vi "H2O_DIAL_NCAR_4CH_v4.05.vi"() -> ()   [LabVIEW 2012]
uses:
  C:/Users/H2ODial/Desktop/Shared Telescope WV DIAL Code/Libraries and VIs/PowerMeterCommands.dll
  Libraries and VIs/PowerMeterCommands.dll
  <vilib>/DAQmx/write.llb/DAQmx Write (Digital 1D Bool NChan 1Samp 1Line).vi
  <vilib>/DAQmx/miscellaneous.llb/DAQmx Fill In Error Info.vi
  <vilib>/Analysis/baseanly.llb/Mean (DBL).vi
  Libraries and VIs/Scalar_Data.vi
  Libraries and VIs/Scalar_Data_3.vi
  Libraries and VIs/Scalar_Data_2.vi
  Libraries and VIs/Scalar_Data_4.vi
  <vilib>/Analysis/NI_AALBase.lvlib
  Libraries and VIs/CLDevIFace.dll
panel:
  out "FileHour":i32=21
  out "L_Count":i32=25
  out "sigma_off_total":dbl[](array[numeric])=[5.235525125067343e-25, 5.206358319245337e-25, 5.177318750524933e-25, 5.148406424862825e-25, 5.119621341127451e-25, 5.090963491196627e-25, 5.062432860011865e-25, 5.034029425635027e-25, 5.005753159352157e-25, 4.977604025706667e-25, 4.949581982592347e-25, 4.921686981325722e-25, 4.893918966711095e-25, 4.866277877122191e-25, 4.8387636445644285e-25, 4.811376194764721e-25, 4.784115447230487e-25, 4.756981315339233e-25, 4.729973706394386e-25, 4.703092521721628e-25, 4.6763376567211625e-25, 4.6497090009594435e-25, 4.623206438225019e-25, 4.596829846622293e-25, 4.57057909862005e-25, 4.544454061150213e-25, 4.518454595652437e-25, 4.492580558158126e-25, 4.4668317993693425e-25, 4.441208164702635e-25, 4.41570949437918e-25, 4.390335623482575e-25, 4.365086382028137e-25, 4.339961595028071e-25, 4.314961082547237e-25, 4.290084659777996e-25, 4.2653321370993085e-25, 4.240703320135042e-25, 4.216198009811418e-25, 4.191816002426457e-25, 4.16755708969195e-25, 4.143421058805604e-25, 4.1194076924960845e-25, 4.095516769084665e-25, 4.0717480625238245e-25, 4.0481013424706545e-25, 4.0245763743206737e-25, 4.001172919260011e-25, 3.977890734322512e-25, 3.9547295724256756e-25, 3.931689182419048e-25, 3.908769309139365e-25, 3.8859696934393876e-25, 3.863290072236815e-25, 3.840730178557474e-25, 3.8182897415734565e-25, 3.7959684866403156e-25, 3.773766135338825e-25, 3.7516824055099053e-25, 3.729717011286995e-25, 3.707869663137923e-25, 3.686140067893342e-25, 3.664527928779591e-25, 3.643032945453827e-25, 3.621654814033011e-25, 3.600393227122229e-25, 3.579247873843723e-25, 3.5582184398664743e-25, 3.5373046074361216e-25, 3.5165060553938904e-25, 3.4958224592064764e-25, 3.475253490990589e-25, 3.454798819536632e-25, 3.4344581103303625e-25, 3.414231025576395e-25, 3.394117224218377e-25, 3.37411636196096e-25, 3.3542280912885406e-25, 3.3344520614845767e-25, 3.3147879186525413e-25, 3.295235305730259e-25, 3.275793862509532e-25, 3.2564632256504646e-25, 3.237243028702917e-25, 3.2181329021119735e-25, 3.1991324732434905e-25, 3.180241366390581e-25, 3.161459202790299e-25, 3.142785600633377e-25, 3.1242201750825597e-25, 3.1057625382770893e-25, 3.0874122993477767e-25, 3.0691690644282785e-25, 3.051032436660927e-25, 3.0330020162078266e-25, 3.0150774002602592e-25, 2.997258183045521e-25, 2.979543955833093e-25, 2.961934306943937e-25, 2.944428821752431e-25, 2.9270270826932477e-25, 2.909728669267514e-25, 2.8925331580414936e-25, 2.875440122654977e-25, 2.8584491338173137e-25, 2.841559759313169e-25, 2.8247715639976386e-25, 2.80808410980223e-25, 2.791496955724979e-25, 2.775009657833479e-25, 2.7586217692567447e-25, 2.742332840183121e-25, 2.7261424178518227e-25, 2.710050046547509e-25, 2.6940552675881075e-25, 2.6781576193155516e-25, 2.6623566370876434e-25, 2.646651853260364e-25, 2.6310427971768174e-25, 2.615528995144771e-25, 2.600109970428841e-25, 2.5847852432207883e-25, 2.569554330624564e-25, 2.554416746633416e-25, 2.5393720020962457e-25, 2.5244196047033826e-25, 2.5095590589459477e-25, 2.4947898660936654e-25, 2.480111524155541e-25, 2.4655235278440513e-25, 2.451025368544176e-25, 2.436616534266772e-25, 2.422296509605852e-25, 2.408064775697375e-25, 2.3939208101763006e-25, 2.3798640871112015e-25, 2.365894076971971e-25, 2.352010246556833e-25, 2.3382120589521406e-25, 2.324498973455175e-25, 2.3108704455300754e-25, 2.2973259267270024e-25, 2.283864864626908e-25, 2.270486702764721e-25, 2.257190880557015e-25, 2.2439768332388837e-25, 2.2308439917739663e-25, 2.2177917827749597e-25, 2.20481962844103e-25, 2.19192694645104e-25, 2.179113149897461e-25, 2.166377647190967e-25, 2.153719841983278e-25, 2.1411391330535246e-25, 2.1286349142540036e-25, 2.1162065743868337e-25, 2.103853497130775e-25, 2.091575060946101e-25, 2.079370638983031e-25, 2.0672395989815037e-25, 2.0551813031976677e-25, 2.0431951082869756e-25, 2.0312803652523447e-25, 2.019436419319984e-25, 2.0076626098781596e-25, 1.9959582703908636e-25, 1.9843227283026113e-25, 1.9727553050009988e-25, 1.9612553156963306e-25, 1.9498220693936616e-25, 1.9384548688025462e-25, 1.9271530103114487e-25, 1.915915783921294e-25, 1.9047424731896738e-25, 1.8936323552292957e-25, 1.8825847006561212e-25, 1.8715987735714719e-25, 1.8606738315918164e-25, 1.8498091257941087e-25, 1.8390039007904753e-25, 1.8282573946936752e-25, 1.8175688392200846e-25, 1.80693745969556e-25, 1.7963624751388698e-25, 1.7858430983630522e-25, 1.7753785360393623e-25, 1.7649679888396773e-25, 1.7546106515613228e-25, 1.7443057132789558e-25, 1.7340523575155863e-25, 1.723849762422857e-25, 1.7136971010131167e-25, 1.7035935413825008e-25, 1.6935382469544605e-25, 1.6835303767796407e-25, 1.6735690858143057e-25, 1.6636535252563445e-25, 1.653782842907513e-25, 1.643956183497921e-25, 1.6341726891478545e-25, 1.624431499756322e-25, 1.6147317534796005e-25, 1.6050725871551994e-25, 1.5954531368896971e-25, 1.585872538492723e-25, 1.576329928151117e-25, 1.566824442883223e-25, 1.5573552212546758e-25, 1.5479214039898043e-25, 1.5385221346219397e-25, 1.5291565602013113e-25, 1.519823831962039e-25, 1.5105231061650234e-25, 1.5012535447460145e-25, 1.49201431624485e-25, 1.482804596459418e-25, 1.4736235693849326e-25, 1.46447042805166e-25, 1.455344375360034e-25, 1.4462446250285657e-25, 1.4371704024629248e-25, 1.4281209456557682e-25, 1.4190955061389853e-25, 1.410093350012645e-25, 1.4011137586880333e-25, 1.3921560301221658e-25, 1.3832194795253431e-25, 1.3743034404767374e-25, 1.3654072658699072e-25, 1.3565303288298996e-25, 1.3476720236918642e-25, 1.3388317669734332e-25, 1.3300089982893968e-25, 1.3212031812258562e-25, 1.3124138043688156e-25, 1.3036403820696332e-25, 1.2948824553577423e-25, 1.2861395928315612e-25, 1.2774113913410786e-25, 1.2686974768684636e-25, 1.2599975053009544e-25, 1.2513111630057894e-25, 1.2426381676023619e-25, 1.2339782685325752e-25, 1.2253312476934588e-25, 1.2166969199403071e-25, 1.2080751335374065e-25, 1.1994657705541538e-25, 1.1908687474046665e-25, 1.182284014933639e-25, 1.1737115587808914e-25, 1.1651513996305814e-25, 1.1566035931942852e-25, 1.1480682304187532e-25, 1.1395454373665928e-25, 1.1310353751750977e-25, 1.1225382399779688e-25, 1.1140542626706877e-25, 1.1055837085176348e-25, 1.097126877076807e-25, 1.0886841014622313e-25, 1.0802557481625692e-25, 1.07184221622742e-25, 1.0634439369229237e-25, 1.0550613727868173e-25, 1.0466950171251473e-25, 1.038345393031225e-25, 1.0300130526116006e-25, 1.0216985760646603e-25, 1.0134025706453978e-25, 1.0051256696943142e-25, 9.968685315566847e-26, 9.886318383691271e-26, 9.804162950309608e-26, 9.722226278487634e-26, 9.640515833439737e-26, 9.559039270504641e-26]
  out "sigma_on_total":dbl[](array[numeric])=[2.04144506552878e-23, 2.03363164868905e-23, 2.025747572591412e-23, 2.017794430211764e-23, 2.009773817105046e-23, 2.0016873309336366e-23, 1.9935365706299817e-23, 1.9853231355693705e-23, 1.977048625166467e-23, 1.9687146378445772e-23, 1.9603227705421816e-23, 1.951874618043596e-23, 1.9433717722469982e-23, 1.9348158215951184e-23, 1.9262083503317138e-23, 1.9175509380334025e-23, 1.9088451588558353e-23, 1.900092581092815e-23, 1.8912947664136064e-23, 1.882453269524831e-23, 1.8735696373998732e-23, 1.8646454089324773e-23, 1.8556821142337575e-23, 1.8466812743522004e-23, 1.837644400527498e-23, 1.8285729940141764e-23, 1.8194685453299388e-23, 1.810332533962471e-23, 1.8011664280533842e-23, 1.7919716836950586e-23, 1.7827497447925897e-23, 1.7735020425748035e-23, 1.7642299952670358e-23, 1.754935007742652e-23, 1.7456184710818656e-23, 1.736281762398895e-23, 1.726926244502896e-23, 1.717553265574508e-23, 1.7081641588579278e-23, 1.6987602425458152e-23, 1.68934281932253e-23, 1.6799131763488586e-23, 1.6704725849056047e-23, 1.6610223002991386e-23, 1.6515635614647057e-23, 1.642097591109307e-23, 1.632625595307178e-23, 1.623148763389859e-23, 1.6136682679517084e-23, 1.6041852645568704e-23, 1.5947008916673987e-23, 1.585216270718842e-23, 1.5757325057977178e-23, 1.5662506836735098e-23, 1.556771873772616e-23, 1.5472971280958616e-23, 1.5378274811478395e-23, 1.5283639499771967e-23, 1.5189075341266753e-23, 1.5094592155613525e-23, 1.5000199588045791e-23, 1.4905907108522535e-23, 1.4811724011961994e-23, 1.471765941921017e-23, 1.4623722277116113e-23, 1.452992135870101e-23, 1.4436265263735662e-23, 1.4342762419712705e-23, 1.4249421083199486e-23, 1.4156249339056498e-23, 1.406325510226225e-23, 1.397044611884901e-23, 1.3877829966903115e-23, 1.378541405732157e-23, 1.3693205635246762e-23, 1.3601211780942827e-23, 1.3509439411338302e-23, 1.3417895281011788e-23, 1.3326585983534608e-23, 1.3235517953452217e-23, 1.3144697466818022e-23, 1.3054130643262744e-23, 1.2963823446919121e-23, 1.287378168942871e-23, 1.2784011028907963e-23, 1.269451697446829e-23, 1.2605304885835775e-23, 1.2516379975894178e-23, 1.2427747311540186e-23, 1.2339411817103151e-23, 1.2251378274123229e-23, 1.2163651324251236e-23, 1.2076235471304545e-23, 1.1989135081970437e-23, 1.190235438818644e-23, 1.1815897489244797e-23, 1.1729768353364932e-23, 1.1643970819286305e-23, 1.1558508598932436e-23, 1.1473385278221191e-23, 1.1388604319479822e-23, 1.1304169063843004e-23, 1.122008273184013e-23, 1.1136348426833785e-23, 1.1052969135364539e-23, 1.0969947730316559e-23, 1.0887286971537587e-23, 1.0804989509475963e-23, 1.07230578850557e-23, 1.0641494533043776e-23, 1.0560301782926725e-23, 1.047948186150434e-23, 1.0399036894250036e-23, 1.031896890763079e-23, 1.0239279830219628e-23, 1.0159971494762414e-23, 1.0081045640686342e-23, 1.0002503914953993e-23, 9.924347874544637e-24, 9.846578987076846e-24, 9.7691986343937e-24, 9.692208112477475e-24, 9.615608634312278e-24, 9.53940133157985e-24, 9.463587255028901e-24, 9.388167378138146e-24, 9.313142597016321e-24, 9.238513733351717e-24, 9.164281535166715e-24, 9.090446678433916e-24, 9.017009769507337e-24, 8.943971345840847e-24, 8.871331877547395e-24, 8.799091769345933e-24, 8.727251362469196e-24, 8.655810934528908e-24, 8.584770703015792e-24, 8.514130824937205e-24, 8.443891399845548e-24, 8.374052469666215e-24, 8.30461402165979e-24, 8.23557598842531e-24, 8.166938250220636e-24, 8.09870063571327e-24, 8.03086292329742e-24, 7.963424843129024e-24, 7.896386077455162e-24, 7.829746261877174e-24, 7.76350498767362e-24, 7.697661801548124e-24, 7.63221620790868e-24, 7.567167669492106e-24, 7.502515609040041e-24, 7.438259409201822e-24, 7.374398415389291e-24, 7.310931935299025e-24, 7.247859240849607e-24, 7.18517956905468e-24, 7.122892123050664e-24, 7.060996072777461e-24, 6.99949055663218e-24, 6.938374681458788e-24, 6.877647524805744e-24, 6.8173081345645e-24, 6.757355530696846e-24, 6.697788705968921e-24, 6.638606626367178e-24, 6.579808233049281e-24, 6.521392441796805e-24, 6.463358144925488e-24, 6.4057042113363034e-24, 6.3484294880639726e-24, 6.291532800599893e-24, 6.23501295336718e-24, 6.178868731199306e-24, 6.123098899483674e-24, 6.067702204884087e-24, 6.01267737674528e-24, 5.958023126645283e-24, 5.903738150186674e-24, 5.849821126538989e-24, 5.7962707201795e-24, 5.743085580692951e-24, 5.6902643436582656e-24, 5.637805631506092e-24, 5.585708053569947e-24, 5.533970207051788e-24, 5.482590677443224e-24, 5.431568039066743e-24, 5.380900855603735e-24, 5.3305876804860644e-24, 5.2806270576492845e-24, 5.231017521895454e-24, 5.1817575992506746e-24, 5.132845807674582e-24, 5.084280657272612e-24, 5.036060650860678e-24, 4.988184284511523e-24, 4.940650047510622e-24, 4.893456423348436e-24, 4.846601889770117e-24, 4.8000849193904994e-24, 4.753903979624906e-24, 4.7080575337261334e-24, 4.662544040368925e-24, 4.617361954873326e-24, 4.572509728567645e-24, 4.5279858098761176e-24, 4.4837886444191376e-24, 4.4399166752196636e-24, 4.396368343110522e-24, 4.353142086723786e-24, 4.310236343387402e-24, 4.267649548693646e-24, 4.225380137567508e-24, 4.1834265436346086e-24, 4.141787200071118e-24, 4.100460539746925e-24, 4.059444995273427e-24, 4.018738999519791e-24, 3.978340985645206e-24, 3.9382493872264135e-24, 3.898462638564106e-24, 3.858979175244214e-24, 3.81979743343543e-24, 3.7809158512434734e-24, 3.742332867827665e-24, 3.704046924201295e-24, 3.666056463311095e-24, 3.628359930032478e-24, 3.590955771418263e-24, 3.553842436936342e-24, 3.517018378534459e-24, 3.480482050624481e-24, 3.444231910627635e-24, 3.4082664187032186e-24, 3.372584038041973e-24, 3.3371832351443385e-24, 3.3020624795514383e-24, 3.2672202442735406e-24, 3.2326550059709053e-24, 3.1983652446833905e-24, 3.164349444235738e-24, 3.130606092186823e-24, 3.0971336800695645e-24, 3.06393070340578e-24, 3.030995661721895e-24, 2.9983270585653876e-24, 2.9659234019996817e-24, 2.933783204123355e-24, 2.9019049814229044e-24, 2.870287254971944e-24, 2.8389285501614312e-24, 2.8078273970940295e-24, 2.7769823303790683e-24, 2.746391889257262e-24, 2.7160546177804717e-24, 2.6859690647949184e-24, 2.65613378374283e-24, 2.6265473332620553e-24, 2.597208276553025e-24, 2.568115182026435e-24, 2.5392666228001165e-24, 2.510661177266997e-24, 2.48229742859929e-24, 2.454173965243289e-24, 2.4262893806011815e-24, 2.3986422732292233e-24, 2.371231246858978e-24, 2.344054910309026e-24, 2.3171118776147202e-24, 2.2904007680434033e-24, 2.2639202059521634e-24, 2.237668821064949e-24, 2.211645248222906e-24, 2.185848127501672e-24, 2.16027610436914e-24]
  out "background start":u32=269
  in  "Tab Control 2":enum32{"WV ND far", "WV ND near"}(tab)
  out "Water Vapor Number Density":dbl[][](graph)=[[1.7566467714554592, 1.7112237483974937, 1.6748749506264644, 1.5531626763016915, 1.4925818532745008, 1.4691395321648246, 1.3246167272218103, 1.2269868164425828, 1.3255222864560143, 1.4516476142332622, 1.4317488856306848, 1.4006762178952012, 1.3734771433422062, 1.3434494748177286, 1.3451253921115185, 1.1715664766487153, 0.9603460494298136, 1.167803410589512, 1.5837995618115461, 1.4928182826946899, 0.7830880837201466, 0.7124646182150762, 1.5821683844017884, 1.897616667905768, 1.3567387444432506, 0.7685875264908889, 0.8821075379606124, 0.9580561941866925, 0.6860769280953256, 0.9548855995658682, 0.34317959293560385, -0.48852203085720447, 0.4000953836211541, 1.6276766516112087, 0.6582217273425924, -0.3701431622041616, 0.5624402493727769, 1.5020315964518778, 1.9490328819529277, 0.5687081180809571, 0.14829866816328646, 0.15078097843341215, -0.4052462468388696, 0.00726247689994212, 0.6405048350399107, 1.070833208753949, 1.2895427721533483, 0.4806362739895196, 1.0023443102054248, 1.0632416785543921, 0.5419834758759072, 1.216133517204536, 2.9403717140528025, 6.026761955773755, 2.4631218194880327, -0.5616309456927226, -2.1863539244969585, -1.1172913943803293, -0.5764679216345628, -0.32669650897300184, 1.367021471278265, 1.8114322755592884, 5.333676793891489, -0.6746298517642445, 0.2493668025284435, -0.968407653253325, -1.2597627805763916, -0.873029286367304, 0.03600152424325076, -0.4128660335725368, -1.9925424606024094, -4.686321918196433, -9.773012324862892, 8.321919527003791, -3.3327600174211867, -2.2694378626967384, -0.7880407452058662, -3.126604726748548, 4.237818794739943, 1.9339834290875324, -0.5031068702025436, 2.834157585206886, 1.9194876875375615, -7.621882484032893, 10.053582111673641, 24.583430974758375, 1.6051353561748916, 1.9018880545441958, -2.199648496161464, -2.8171837647098044, -0.1810860182335741, -5.818897288164005, -5.390599800188094, -5.557229048352483, -11.486454195723043, -1.7389583913430502, 10.399164750341773, -1.6277519987253517, -10.371881860352497, -4.1738257491608035, 4.726765211939229, 3.4342788042530907, 1.9890722023134209, 2.4803275304917283, -3.41607671638549, -21.568626510054933, 3.388736921345587, 1.9568309789098535, -4.193155315940581, -5.703648396321129, -9.41827741518324, -0.21393347906320512, 19.9442339598812, -7.779013774001198, -17.279927512309417, -1.0627832528431156, -5.628901623765271, -15.970763810695905, -4.961662952263955, -10.607717740119206, -6.080359409806072, -4.630196687396562, -15.179266411863631, 16.998783731568285, 19.683522058787823, 4.441696343538448, 2.9936653651043224, 10.18325033335466, 12.243607901212322, 21.965007450796293, -11.495554392257876, -8.606917738950113, 1.0275123216560922, 43.36786043195841, 3.9650450738050127, -6.739703774348581, -inf, nan, nan, nan, nan, nan, nan, nan, nan, nan, inf, 13.30350327244809, -6.9195038865649385, -30.02574288642436, 29.98478311978834, 27.14478668914213, -11.656702325292523, -15.57129494579555, 15.10678922185829, -47.07881448032253, -7.481444647178393, -23.95171395849395, 6.309430158448025, 35.89025473241871, 11.91244899569984, 0.8006492734233216, 11.615817365890178, -11.047456747490754, -15.125295235644119, 39.29548202856169, -9.353666557107148, 6.280426361037719, 22.81560033773844, 32.07648611690262, -11.533089659843613, -2.3579814912048973, 0.3834128869563981, 21.166755898932436, -9.305881096161668, -22.47653352972326, -1.3457820555854025, 8.047662763912756, -9.543851204922277, -12.776458583854794, -10.529162622965355, -24.75070784542627, -49.21697297753648, -15.586326392775408, 27.997138034650167, 11.10292972403797, 9.130712531006333, 7.442724853607613, 0.5164059061518099, -25.4542678895718, 15.365380043788852, 7.940212369868569, 34.78339739007152, -44.476237527262874, -13.559779658265485, -7.993736080670773, 8.358804396451996, -0.45638812899210496, 1.012789493341061, -0.903707718634473, -5.80247336277099, 37.864941956157445, 33.65331183466617, 66.59566921633602, 4.954744530886738, -1.8216197646865204, -21.762498368841232, 69.36941467993034, 21.43158181763081, 23.944428219537183, -0.9467901008841881, -35.80343613723175, -18.906417630181103, -28.075372073073307, -22.003823523938692, 10.913121198905674, 23.828352681206827, -99.37444975983206, -12.444806194392113, -10.785166308820509, -13.026219509633277, 2.473570893883758, 21.774065449921164, 32.49619526466478, -30.524578490924462, -39.86007255504935, 2.3214561755513548, 20.741356086607233, -5.241565693386122, 47.45719238471328, 6.638705375973361, 14.532285527708414, -29.84211791164372, -33.815878650101176, 120.87936843977374, 6.853660622102851, -117.08570912517183, -11.080618171015148, -53.60576388696484, -129.46751362308734, 17.645695728779145, -69.93848547258612, -26.734733036250308, -13.272282442538005, -123.61198307600142, 18.994451307979766, 119.20062246758617, 5.331441778858514, 26.027221748727683, 46.079407834078616, 21.785832764745205, 77.36529322409149, 31.088969869188524, 21.848530603867186, 74.54553200715928, -27.475237169504652, 52.95613566614017, -47.73571888711182, 79.6344255893079, -14.920185717589504, -48.18901915049144, -24.773698129219312, -3.7504985766762235, -4.013672684158284, 3.8346346175193293, 41.18401135017199, -76.98669890147586, 69.94729966645377, -83.44853618010815, 60.39596177960426, 59.04178017636866, 50.787618001797405, 48.09534192486351, 47.39622772647818, 4.438710312021304, 39.06355265414693, 0.0, 0.0, 0.0, 0.0]]
  out "Water Vapor Number Density 2":dbl[][](graph)=[[nan, nan, nan, nan, nan, nan, nan, nan, nan, nan, nan, nan, nan, nan, nan, nan, nan, nan, nan, nan, nan, nan, nan, nan, nan, nan, nan, nan, nan, nan, nan, nan, nan, nan, nan, nan, nan, nan, nan, nan, nan, nan, nan, nan, nan, nan, nan, nan, nan, nan, nan, nan, nan, nan, nan, nan, nan, nan, nan, nan, nan, nan, nan, nan, nan, nan, nan, nan, nan, nan, nan, nan, nan, nan, nan, nan, nan, nan, nan, nan, nan, nan, nan, nan, nan, nan, nan, nan, nan, nan, nan, nan, nan, nan, nan, nan, nan, nan, nan, nan, nan, nan, nan, nan, nan, nan, nan, nan, nan, nan, nan, nan, nan, nan, nan, nan, nan, nan, nan, nan, nan, nan, nan, nan, nan, nan, nan, nan, nan, nan, nan, nan, nan, nan, nan, nan, nan, nan, nan, nan, nan, nan, nan, nan, nan, nan, nan, nan, nan, nan, nan, nan, nan, nan, nan, nan, nan, nan, nan, nan, nan, nan, nan, nan, nan, nan, nan, nan, nan, nan, nan, nan, nan, nan, nan, nan, nan, nan, nan, nan, nan, nan, nan, nan, nan, nan, nan, nan, nan, nan, nan, nan, nan, nan, nan, nan, nan, nan, nan, nan, nan, nan, nan, nan, nan, nan, nan, nan, nan, nan, nan, nan, nan, nan, nan, nan, nan, nan, nan, nan, nan, nan, nan, nan, nan, nan, nan, nan, nan, nan, nan, nan, nan, nan, nan, nan, nan, nan, nan, nan, nan, nan, nan, nan, nan, nan, nan, nan, nan, nan, nan, nan, nan, nan, nan, nan, nan, nan, nan, nan, nan, nan, nan, nan, nan, nan, nan, nan, nan, nan, nan, nan, nan, nan, nan, nan, 0.0, 0.0, 0.0, 0.0]] caption="Water Vapor Number Density"
  out "RingBuffer offline near":dbl[][](array[numeric])
  out "RingBuffer aerosol near":dbl[][](array[numeric])
  in  "?":T1(tab)=enum."Raw Counts far"
  out "NRB":dbl[][](graph)=[[9.476976335603298e-05, 0.0005753128498656646, 0.0016970306725621529, 0.0035534832971788476, 0.006071721053046345, 0.008970749768071643, 0.01200847035901779, 0.015038193264303132, 0.017834981927160792, 0.020360035071458532, 0.022746015449932717, 0.025016125530806687, 0.02719241788441539, 0.02933837894016536, 0.03125755534620425, 0.032709549671793355, 0.03410397874989958, 0.03547363015805232, 0.036657591394332875, 0.0378690817139413, 0.03917814075997203, 0.04025679874994388, 0.04089491970302044, 0.041837532857835445, 0.042185448900406514, 0.041613971578980204, 0.04142285738950741, 0.04126487099656473, 0.04043148675558985, 0.03756869921461678, 0.03245079866111025, 0.027946371031990117, 0.024967022232250023, 0.022538693033476637, 0.020988486697919435, 0.020355378441952433, 0.019106590793189878, 0.018553649002290496, 0.01797850487900519, 0.01702933408875092, 0.017234825206185297, 0.016245558602627972, 0.015099608574420302, 0.014412793306488862, 0.013769073244293169, 0.013250389553255347, 0.012940166117206513, 0.012397757444172597, 0.012189906348387756, 0.012362011844732134, 0.01135744245014516, 0.011139035595917914, 0.010193813217974013, 0.008211699408749069, 0.00828695956983334, 0.008653028642202146, 0.00768848813101233, 0.007944003516039203, 0.009407158642137347, 0.010137900504628481, 0.010331548861359268, 0.008802094202070973, 0.008107736160050491, 0.008043343325181558, 0.006913621323094165, 0.006218641761016856, 0.00608136087759757, 0.006429888062849834, 0.00520310435058665, 0.004580297994030712, 0.006623685652882607, 0.007311049308142974, 0.006067397494135996, 0.006491798233211616, 0.006807399111558534, 0.0058842864618796455, 0.004905025645619411, 0.004740179123447561, 0.0051939762897226065, 0.004954761339962726, 0.004795766571469106, 0.005205596132798339, 0.004201634139811345, 0.0037457138020616787, 0.00529004181764211, 0.004465179855272384, 0.005336236420925891, 0.006282216542213424, 0.004772353935915863, 0.00452003001981128, 0.005204046490786279, 0.005496773942817911, 0.005969454324061356, 0.0061421754750257095, 0.007076167043858164, 0.005575349859747556, 0.003542137313518651, 0.0036511341669561203, 0.00470657935472985, 0.00772946288539167, 0.007355627137890949, 0.006075588196503905, 0.006090471534399443, 0.006075713294560285, 0.005103717459911745, 0.0046879075252070895, 0.004635365170749996, 0.0028927838186322916, 0.005294533151855598, 0.00811217310614376, 0.00590150094704256, 0.0050632051063556945, 0.005437909212564243, 0.0043467494178044365, 0.0013851405304458764, 0.003004821937200342, 0.006708915105310044, 0.009197445944443085, 0.007709839718149087, 0.0023619129515158386, -0.000799268290397213, 0.00297441876999425, 0.0034531592804808242, -0.0019408528592538105, -0.0003319316142057259, -0.0031020209709489775, -0.004685331128153522, 0.005904891382068294, 0.015000275609983344, 0.00936805783132079, 0.001161514990141057, 0.0013084382693883373, 0.0049550910904123235, 0.007691243063106685, 0.008977008540048617, 0.0035363281596428363, -0.0005378103269298039, -0.0035798935458200135, 0.0011883941537936358, 0.008225970516181846, 0.007656344140856141, 0.005075580170439123, -0.0006869749676299755, 0.0014547053346970623, 0.006071359789051531, 0.005576178405811973, 7.472970524046106e-05, -0.0014392440608992307, 0.004409227368747632, 0.009137382320870916, 0.003936992021506711, 0.002048866441916494, 0.008783701563844535, 0.00881101926132704, 0.0017744605782389071, -0.0015990432553891377, 0.007239635457859621, 0.010600536203863014, 0.0006494691594315171, 0.0029658234762455927, 0.00921401984925274, -0.002340271303637164, -0.013394918543133849, -0.004225446660139794, 0.0062476694016030225, 0.005200478128375437, 0.006262261212075584, 0.002746925988792983, 0.007647822255329004, 0.007381646854046047, 0.00486839127937324, 0.00028500479763016634, -0.002262261694663059, -0.001391044931209939, 0.005968798886761723, 0.014148180121976774, -0.004264089420036615, -0.0028645080376568785, 0.009727330081072131, 0.00515423373409494, 0.0035526631679868824, -0.002012831156920732, -0.0069984113452448505, 0.002333305127234436, 0.01165853729791182, 0.011229419906661446, 0.0019781087762913967, 0.002916044077523569, 0.0025500763264635893, -0.007410290132612892, -0.016679991350251312, -0.013167251562984691, -0.005023836001253541, -0.011862582247623182, -0.018278237845436075, -0.012582894560523722, -0.009068805512834146, -0.002237030406289816, -0.004069379818483554, 0.0021144877601388646, 0.02124747345054341, 0.015310784681580264, 0.010016634922605122, 0.00528391879853587, -0.00888604211747558, -0.006509594206171102, 0.008192480823558385, 0.002180159189879256, 0.00705673151599474, 0.0179637388053101, 0.019894894548171907, 0.014033133357429136, -0.008864675575143878, -0.0036312966149882634, 0.015689170217100406, 0.010879626802485462, 0.010573474065596729, 0.019593268736771936, 0.002298377099526465, -0.011250232706638474, -0.0030885450015696574, 0.005892286625456142, -0.003206118965745949, -0.005713806319119231, -0.0007002987173920376, -0.0017789588354741833, -0.00020365830930791864, -0.0022600191621767003, 0.015791025552977036, 0.010832887109405664, -0.009108137668699516, -0.006129223360177645, -0.0015556068431292088, 0.003300297413580269, 0.0046927360612964136, 0.0015684108743274146, 0.0022754732753808623, 0.010270310803552203, 0.007887520143392869, -0.005492102811724082, -0.006398785622739085, 0.00960576875642872, -0.005338541065383191, -0.01567699604612269, -0.0033509670373703553, -0.0038268337936362765, -0.0011453485802606202, -0.0006988621233230238, -0.004609930948182576, 0.00886185918558943, 0.01165635959194438, 0.0021020205237233763, 0.0041742320835957926, 0.00261362021461076, 0.0010279952563537712, 0.0002266410274718338, -0.01755514686518196, -0.020569414496907742, -0.0002651245521295679, 0.0013191817257425771, -0.014151548188129337, -0.003916914478353181, 0.020059267474150624, -0.0038908621180602132, -0.018578352080135096, -0.015048502477482188, -0.0032754063317817867, 0.007611306333458159, -0.00046473812629934915, -0.010012222000579307, -0.01707083347537678, -0.004587129190427817, 0.00845026692989676, 0.002948692111647269, -0.002633991736485534, 0.01550527129308583, 0.02007199253610184, 0.0, 0.0, 0.0]] caption="Water Vapor Number Density"
  out "NRB 2":dbl[][](graph) caption="Water Vapor Number Density"
  out "raw counts":dbl[][](graph)=[[363.2, 635.2, 978.2, 1144.2, 1306.2, 1380.2, 1401.2, 1308.2, 1288.2, 1183.2, 1050.2, 998.2, 994.2, 897.2, 874.2, 669.2, 612.2, 614.2, 555.2, 505.2, 484.2, 509.2, 433.2, 399.2, 417.2, 326.2, 320.2, 293.2, 268.2, 283.2, 171.2, 162.2, 156.2, 130.2, 70.19999999999999, 100.19999999999999, 62.19999999999999, 27.19999999999999, 41.19999999999999, 1.1999999999999886, 54.19999999999999, 43.19999999999999, 21.19999999999999, 24.19999999999999, 39.19999999999999, 22.19999999999999, 25.19999999999999, 39.19999999999999, 21.19999999999999, 30.19999999999999, 20.19999999999999, 0.19999999999998863, -6.800000000000011, 5.199999999999989, -16.80000000000001, -18.80000000000001, 17.19999999999999, -13.800000000000011, 6.199999999999989, 28.19999999999999, 17.19999999999999, 21.19999999999999, 24.19999999999999, -0.8000000000000114, 2.1999999999999886, 26.19999999999999, 7.199999999999989, 8.199999999999989, -7.800000000000011, -13.800000000000011, -16.80000000000001, -18.80000000000001, 3.1999999999999886, -11.800000000000011, 18.19999999999999, -4.800000000000011, -9.800000000000011, 8.199999999999989, 22.19999999999999, -4.800000000000011, 6.199999999999989, 7.199999999999989, -14.800000000000011, -8.800000000000011, -18.80000000000001, -3.8000000000000114, -8.800000000000011, -21.80000000000001, -10.800000000000011, -27.80000000000001, -2.8000000000000114, 2.1999999999999886, -21.80000000000001, -16.80000000000001, 14.199999999999989, 2.1999999999999886, 20.19999999999999, -26.80000000000001, -16.80000000000001, -9.800000000000011, -34.80000000000001, -0.8000000000000114, -0.8000000000000114, -23.80000000000001, -4.800000000000011, -19.80000000000001, -7.800000000000011, 7.199999999999989, -7.800000000000011, 20.19999999999999, -0.8000000000000114, 1.1999999999999886, 1.1999999999999886, 2.1999999999999886, 13.199999999999989, 1.1999999999999886, -18.80000000000001, 10.199999999999989, 13.199999999999989, 0.19999999999998863, -12.800000000000011, -3.8000000000000114, -8.800000000000011, 8.199999999999989, -27.80000000000001, -9.800000000000011, 2.1999999999999886, 1.1999999999999886, -8.800000000000011, 12.199999999999989, 2.1999999999999886, -11.800000000000011, -17.80000000000001, 0.19999999999998863, -7.800000000000011, -17.80000000000001, 16.19999999999999, -16.80000000000001, -18.80000000000001, -15.800000000000011, -9.800000000000011, 18.19999999999999, 5.199999999999989, 4.199999999999989, -20.80000000000001, 7.199999999999989, 17.19999999999999, -2.8000000000000114, -16.80000000000001, -13.800000000000011, -20.80000000000001, -27.80000000000001, -9.800000000000011, -3.8000000000000114, -29.80000000000001, -24.80000000000001, -3.8000000000000114, -3.8000000000000114, -7.800000000000011, -5.800000000000011, 13.199999999999989, -6.800000000000011, -30.80000000000001, 10.199999999999989, 9.199999999999989, -4.800000000000011, -1.8000000000000114, 4.199999999999989, -1.8000000000000114, 6.199999999999989, -12.800000000000011, -9.800000000000011, -12.800000000000011, -20.80000000000001, 20.19999999999999, -7.800000000000011, -17.80000000000001, -3.8000000000000114, -15.800000000000011, -2.8000000000000114, -11.800000000000011, -4.800000000000011, -3.8000000000000114, -15.800000000000011, 0.19999999999998863, -1.8000000000000114, -1.8000000000000114, -22.80000000000001, -5.800000000000011, -6.800000000000011, 1.1999999999999886, 2.1999999999999886, 11.199999999999989, 19.19999999999999, -4.800000000000011, 11.199999999999989, -12.800000000000011, -19.80000000000001, 1.1999999999999886, -15.800000000000011, -8.800000000000011, -4.800000000000011, -10.800000000000011, -8.800000000000011, -12.800000000000011, -9.800000000000011, -3.8000000000000114, -22.80000000000001, -26.80000000000001, -32.80000000000001, 9.199999999999989, -9.800000000000011, -13.800000000000011, 7.199999999999989, 12.199999999999989, -12.800000000000011, 4.199999999999989, 0.19999999999998863, -10.800000000000011, 12.199999999999989, -6.800000000000011, -4.800000000000011, -0.8000000000000114, -8.800000000000011, 4.199999999999989, -4.800000000000011, 1.1999999999999886, 10.199999999999989, 1.1999999999999886, -23.80000000000001, -8.800000000000011, -6.800000000000011, -30.80000000000001, -15.800000000000011, 10.199999999999989, -14.800000000000011, 12.199999999999989, 9.199999999999989, 4.199999999999989, 11.199999999999989, 3.1999999999999886, -0.8000000000000114, 10.199999999999989, -5.800000000000011, -10.800000000000011, -18.80000000000001, -27.80000000000001, -33.80000000000001, 1.1999999999999886, -12.800000000000011, -26.80000000000001, -20.80000000000001, -14.800000000000011, -16.80000000000001, 1.1999999999999886, -24.80000000000001, 3.1999999999999886, -16.80000000000001, -4.800000000000011, -12.800000000000011, -8.800000000000011, -27.80000000000001, -19.80000000000001, -13.800000000000011, -20.80000000000001, 12.199999999999989, -0.8000000000000114, 6.199999999999989, 0.19999999999998863, -2.8000000000000114, 3.1999999999999886, -1.8000000000000114, 18.19999999999999, -16.80000000000001, -12.800000000000011, 9.199999999999989, 6.199999999999989, -8.800000000000011, 6.199999999999989, 0.0]] caption="Water Vapor Number Density"
  out "raw counts near":dbl[][](graph) caption="Water Vapor Number Density"
  out "Aerosol Smoothed 2":dbl[](array[numeric])
  out "Off-Line Smoothed 2":dbl[](array[numeric])
  out "Off-Line Bin Readings 2":dbl[](array[numeric])
  out "On-Line Smoothed 2":dbl[](array[numeric])
  out "On-Line Bin Readings 2":dbl[](array[numeric])
  in  "stop":bool
  in  "Reset Average":bool=TRUE
  in  "Save Data?":bool=TRUE
  in  "Collect Data?":bool=TRUE
  in  "ILX Address":i32=6 min=0 step=1
  in  "Lambda On DBR Current":dbl=169.69
  in  "Lambda Off DBR Current":dbl=172.7499999999999
  in  "Tab Control":T2(tab)=enum."g/m^3"
  out "Water Vapor Number Density  2":cluster{"Y":dbl[], "Y":dbl[]}[](graph)=[{"Y"=array[276 elements], "Y"=array[280 elements]}, {"Y"=[nan, nan, nan, nan, nan, nan, nan, nan, nan, nan, nan, nan, nan, nan, nan, nan, nan, nan, nan, nan, nan, nan, nan, nan, nan, nan, nan, nan, nan, nan, nan, nan, nan, nan, nan, nan, nan, nan, nan, nan, nan, nan, nan, nan, nan, nan, nan, nan, nan, nan, nan, nan, nan, nan, nan, nan, nan, nan, nan, nan, nan, nan, nan, nan, nan, nan, nan, nan, nan, nan, nan, nan, nan, nan, nan, nan, nan, nan, nan, nan, nan, nan, nan, nan, nan, nan, nan, nan, nan, nan, nan, nan, nan, nan, nan, nan, nan, nan, nan, nan, nan, nan, nan, nan, nan, nan, nan, nan, nan, nan, nan, nan, nan, nan, nan, nan, nan, nan, nan, nan, nan, nan, nan, nan, nan, nan, nan, nan, nan, nan, nan, nan, nan, nan, nan, nan, nan, nan, nan, nan, nan, nan, nan, nan, nan, nan, nan, nan, nan, nan, nan, nan, nan, nan, nan, nan, nan, nan, nan, nan, nan, nan, nan, nan, nan, nan, nan, nan, nan, nan, nan, nan, nan, nan, nan, nan, nan, nan, nan, nan, nan, nan, nan, nan, nan, nan, nan, nan, nan, nan, nan, nan, nan, nan, nan, nan, nan, nan, nan, nan, nan, nan, nan, nan, nan, nan, nan, nan, nan, nan, nan, nan, nan, nan, nan, nan, nan, nan, nan, nan, nan, nan, nan, nan, nan, nan, nan, nan, nan, nan, nan, nan, nan, nan, nan, nan, nan, nan, nan, nan, nan, nan, nan, nan, nan, nan, nan, nan, nan, nan, nan, nan, nan, nan, nan, nan, nan, nan, nan, nan, nan, nan, nan, nan, nan, nan, nan, nan, nan, nan, nan, nan, nan, nan, nan, nan], "Y"=array[280 elements]}]
  out "Absolute Humidity":cluster{"Y":dbl[], "Y":dbl[]}[](graph)=[{"Y"=array[276 elements], "Y"=array[280 elements]}, {"Y"=[nan, nan, nan, nan, nan, nan, nan, nan, nan, nan, nan, nan, nan, nan, nan, nan, nan, nan, nan, nan, nan, nan, nan, nan, nan, nan, nan, nan, nan, nan, nan, nan, nan, nan, nan, nan, nan, nan, nan, nan, nan, nan, nan, nan, nan, nan, nan, nan, nan, nan, nan, nan, nan, nan, nan, nan, nan, nan, nan, nan, nan, nan, nan, nan, nan, nan, nan, nan, nan, nan, nan, nan, nan, nan, nan, nan, nan, nan, nan, nan, nan, nan, nan, nan, nan, nan, nan, nan, nan, nan, nan, nan, nan, nan, nan, nan, nan, nan, nan, nan, nan, nan, nan, nan, nan, nan, nan, nan, nan, nan, nan, nan, nan, nan, nan, nan, nan, nan, nan, nan, nan, nan, nan, nan, nan, nan, nan, nan, nan, nan, nan, nan, nan, nan, nan, nan, nan, nan, nan, nan, nan, nan, nan, nan, nan, nan, nan, nan, nan, nan, nan, nan, nan, nan, nan, nan, nan, nan, nan, nan, nan, nan, nan, nan, nan, nan, nan, nan, nan, nan, nan, nan, nan, nan, nan, nan, nan, nan, nan, nan, nan, nan, nan, nan, nan, nan, nan, nan, nan, nan, nan, nan, nan, nan, nan, nan, nan, nan, nan, nan, nan, nan, nan, nan, nan, nan, nan, nan, nan, nan, nan, nan, nan, nan, nan, nan, nan, nan, nan, nan, nan, nan, nan, nan, nan, nan, nan, nan, nan, nan, nan, nan, nan, nan, nan, nan, nan, nan, nan, nan, nan, nan, nan, nan, nan, nan, nan, nan, nan, nan, nan, nan, nan, nan, nan, nan, nan, nan, nan, nan, nan, nan, nan, nan, nan, nan, nan, nan, nan, nan, nan, nan, nan, nan, nan, nan], "Y"=array[280 elements]}]
  out "NRB plot":cluster{"Y":dbl[], "Y":dbl[]}[](graph)
  in  "background length":i32=10
  out "Correction":cluster{"Y":dbl[], "Y":dbl[]}[](graph)=[{"Y"=array[277 elements], "Y"=array[280 elements]}, {"Y"=[1.0, 1.0, 1.0, 1.0, 1.0, 1.0, 1.0, 1.0, 1.0, 1.0, 1.0, 1.0, 1.0, 1.0, 1.0, 1.0, 1.0, 1.0, 1.0, 1.0, 1.0, 1.0, 1.0, 1.0, 1.0, 1.0, 1.0, 1.0, 1.0, 1.0, 1.0, 1.0, 1.0, 1.0, 1.0, 1.0, 1.0, 1.0, 1.0, 1.0, 1.0, 1.0, 1.0, 1.0, 1.0, 1.0, 1.0, 1.0, 1.0, 1.0, 1.0, 1.0, 1.0, 1.0, 1.0, 1.0, 1.0, 1.0, 1.0, 1.0, 1.0, 1.0, 1.0, 1.0, 1.0, 1.0, 1.0, 1.0, 1.0, 1.0, 1.0, 1.0, 1.0, 1.0, 1.0, 1.0, 1.0, 1.0, 1.0, 1.0, 1.0, 1.0, 1.0, 1.0, 1.0, 1.0, 1.0, 1.0, 1.0, 1.0, 1.0, 1.0, 1.0, 1.0, 1.0, 1.0, 1.0, 1.0, 1.0, 1.0, 1.0, 1.0, 1.0, 1.0, 1.0, 1.0, 1.0, 1.0, 1.0, 1.0, 1.0, 1.0, 1.0, 1.0, 1.0, 1.0, 1.0, 1.0, 1.0, 1.0, 1.0, 1.0, 1.0, 1.0, 1.0, 1.0, 1.0, 1.0, 1.0, 1.0, 1.0, 1.0, 1.0, 1.0, 1.0, 1.0, 1.0, 1.0, 1.0, 1.0, 1.0, 1.0, 1.0, 1.0, 1.0, 1.0, 1.0, 1.0, 1.0, 1.0, 1.0, 1.0, 1.0, 1.0, 1.0, 1.0, 1.0, 1.0, 1.0, 1.0, 1.0, 1.0, 1.0, 1.0, 1.0, 1.0, 1.0, 1.0, 1.0, 1.0, 1.0, 1.0, 1.0, 1.0, 1.0, 1.0, 1.0, 1.0, 1.0, 1.0, 1.0, 1.0, 1.0, 1.0, 1.0, 1.0, 1.0, 1.0, 1.0, 1.0, 1.0, 1.0, 1.0, 1.0, 1.0, 1.0, 1.0, 1.0, 1.0, 1.0, 1.0, 1.0, 1.0, 1.0, 1.0, 1.0, 1.0, 1.0, 1.0, 1.0, 1.0, 1.0, 1.0, 1.0, 1.0, 1.0, 1.0, 1.0, 1.0, 1.0, 1.0, 1.0, 1.0, 1.0, 1.0, 1.0, 1.0, 1.0, 1.0, 1.0, 1.0, 1.0, 1.0, 1.0, 1.0, 1.0, 1.0, 1.0, 1.0, 1.0, 1.0, 1.0, 1.0, 1.0, 1.0, 1.0, 1.0, 1.0, 1.0, 1.0, 1.0, 1.0, 1.0, 1.0, 1.0, 1.0, 1.0, 1.0, 1.0, 1.0, 1.0, 1.0, 1.0, 1.0, 1.0, 1.0, 1.0, 1.0, 1.0, 1.0, 1.0, 1.0, 1.0, 1.0, 1.0, 1.0, 1.0], "Y"=array[280 elements]}]
  in  "dead time":dbl=3.7e-08
  out "Optical Depth":cluster{"Y":dbl[], "Y":dbl[]}[](graph) caption="XY Graph"
  out "RingBuffer offline far":dbl[][](array[numeric])
  out "RingBuffer aerosol far":dbl[][](array[numeric])
  in  "Weather":T3(tab)=enum."Pulse Energy (Micro Joule)"
  in  "Temperature (C)":dbl=15.0
  out "Temperature (C)":dbl(graph)=15.0
  in  "Pressure (mbar or hPa)":dbl=832.0
  out "Pressure (mb)":dbl(graph)=832.0
  out "Relative Humdity (%)":dbl(graph)=40.0
  out "Pulse Energy (Micro Joule)":T4(graph)={"Online Pulse Energy"=3.2240871428571425, "Pulse Energy Offline"=3.2413214285714282}
  out "?":cluster{"mean":dbl, "mean":dbl}(graph)={"mean"=33760.0, "mean"=0.0}
  out "Index":i32=26
  out "Aerosol Smoothed":dbl[](array[numeric])=[502.92631578947373, 761.8013157894738, 996.9723684210527, 1172.7355263157892, 1281.3999999999996, 1314.4131578947367, 1292.9065789473682, 1240.1171052631578, 1162.7486842105263, 1075.867105263158, 993.9526315789474, 919.0644736842105, 851.663157894737, 792.6434210526318, 735.9592105263159, 677.1828947368422, 625.6697368421054, 580.6894736842107, 538.7355263157896, 502.41315789473697, 471.5644736842106, 441.5973684210527, 410.5315789473685, 385.79473684210535, 358.5776315789475, 327.11052631578957, 301.9921052631579, 279.7815789473684, 255.59736842105264, 221.98552631578946, 179.63026315789472, 145.2157894736842, 122.01184210526314, 103.77499999999999, 91.20263157894736, 83.61052631578946, 74.30131578947368, 68.40657894736843, 62.932894736842115, 56.66973684210526, 54.59078947368421, 49.038157894736855, 43.485526315789485, 39.643421052631595, 36.2092105263158, 33.34736842105264, 31.196052631578958, 28.65657894736843, 27.038157894736848, 26.334210526315793, 23.255263157894742, 21.939473684210533, 19.32763157894737, 14.998684210526315, 14.590789473684211, 14.696052631578945, 12.60394736842105, 12.577631578947363, 14.393421052631576, 14.998684210526314, 14.78815789473684, 12.196052631578944, 10.880263157894731, 10.459210526315786, 8.715789473684211, 7.6039473684210535, 7.215789473684212, 7.406578947368421, 5.821052631578946, 4.978947368421053, 6.998684210526314, 7.511842105263156, 6.064473684210526, 6.314473684210525, 6.446052631578946, 5.426315789473685, 4.406578947368422, 4.15, 4.432894736842105, 4.123684210526315, 3.8934210526315782, 4.123684210526315, 3.2486842105263163, 2.8276315789473685, 3.8999999999999995, 3.2157894736842105, 3.7552631578947375, 4.321052631578948, 3.2092105263157897, 2.9723684210526318, 3.347368421052632, 3.4592105263157906, 3.6763157894736853, 3.702631578947369, 4.1763157894736835, 3.2223684210526313, 2.005263157894737, 2.0250000000000004, 2.5578947368421057, 4.117105263157894, 3.8407894736842105, 3.1105263157894742, 3.0578947368421057, 2.992105263157895, 2.465789473684211, 2.2223684210526318, 2.1565789473684216, 1.3210526315789477, 2.373684210526316, 3.5710526315789473, 2.5513157894736844, 2.1500000000000004, 2.2684210526315796, 1.7815789473684216, 0.5578947368421058, 1.1894736842105267, 2.610526315789474, 3.51842105263158, 2.900000000000001, 0.8736842105263162, -0.29078947368421015, 1.0644736842105265, 1.2157894736842108, -0.6723684210526312, -0.11315789473684168, -1.04078947368421, -1.547368421052631, 1.9197368421052632, 4.8013157894736835, 2.9526315789473685, 0.36052631578947414, 0.40000000000000047, 1.4921052631578953, 2.2815789473684216, 2.6236842105263163, 1.0184210526315793, -0.15263157894736798, -1.0013157894736837, 0.32763157894736894, 2.2355263157894742, 2.0513157894736844, 1.3407894736842108, -0.1789473684210522, 0.3736842105263163, 1.5381578947368426, 1.3934210526315796, 0.018421052631579393, -0.34999999999999953, 1.0578947368421059, 2.163157894736843, 0.9197368421052641, 0.47236842105263205, 1.9986842105263163, 1.978947368421053, 0.3934210526315794, -0.34999999999999953, 1.5644736842105265, 2.261842105263158, 0.13684210526315838, 0.617105263157895, 1.8934210526315793, -0.4749999999999994, -2.685526315789473, -0.8368421052631574, 1.2223684210526322, 1.0052631578947373, 1.196052631578948, 0.5184210526315794, 1.4263157894736844, 1.3605263157894738, 0.8868421052631583, 0.05131578947368465, -0.4026315789473679, -0.2447368421052626, 1.0381578947368424, 2.4328947368421057, -0.7249999999999996, -0.48157894736842066, 1.6171052631578953, 0.8473684210526321, 0.5776315789473689, -0.32368421052631524, -1.1131578947368417, 0.36710526315789516, 1.8144736842105267, 1.728947368421053, 0.30131578947368465, 0.43947368421052674, 0.3802631578947373, -1.0934210526315786, -2.435526315789473, -1.902631578947368, -0.7184210526315785, -1.678947368421052, -2.560526315789473, -1.744736842105263, -1.2447368421052627, -0.3039473684210522, -0.5473684210526312, 0.2815789473684215, 2.8013157894736844, 1.9986842105263163, 1.2947368421052636, 0.6763157894736846, -1.1263157894736837, -0.8171052631578942, 1.0184210526315793, 0.26842105263157945, 0.8605263157894737, 2.169736842105263, 2.3802631578947375, 1.6631578947368428, -1.04078947368421, -0.4223684210526311, 1.8078947368421057, 1.2421052631578953, 1.196052631578948, 2.196052631578948, 0.2552631578947373, -1.2381578947368417, -0.33684210526315744, 0.6368421052631583, -0.34342105263157846, -0.6065789473684206, -0.07368421052631535, -0.18552631578947323, -0.02105263157894692, -0.2315789473684206, 1.6039473684210535, 1.0907894736842114, -0.909210526315789, -0.6065789473684207, -0.15263157894736795, 0.3210526315789478, 0.45263157894736883, 0.1500000000000004, 0.21578947368421098, 0.965789473684211, 0.7355263157894741, -0.5078947368421048, -0.5868421052631574, 0.8736842105263163, -0.48157894736842055, -1.402631578947368, -0.29736842105263117, -0.33684210526315744, -0.09999999999999953, -0.060526315789473234, -0.39605263157894693, 0.7552631578947373, 0.9855263157894741, 0.17631578947368465, 0.347368421052632, 0.21578947368421098, 0.08421052631578993, 0.018421052631579393, -1.41578947368421, -1.646052631578947, -0.021052631578946934, 0.1039473684210531, -1.1065789473684207, -0.3039473684210522, 1.5447368421052636, -0.29736842105263117, -1.409210526315789, -1.1328947368421047, -0.2447368421052627, 0.5644736842105268, -0.034210526315789025, -0.7315789473684207, -1.2381578947368417, -0.3302631578947364, 0.6039473684210531, 0.20921052631578996, -0.18552631578947326, 1.08421052631579, 1.3934210526315793]
  out "Off-Line  Bin Readings":dbl[](array[numeric])=[532.0, 804.0, 1147.0, 1313.0, 1475.0, 1549.0, 1570.0, 1477.0, 1457.0, 1352.0, 1219.0, 1167.0, 1163.0, 1066.0, 1043.0, 838.0, 781.0, 783.0, 724.0, 674.0, 653.0, 678.0, 602.0, 568.0, 586.0, 495.0, 489.0, 462.0, 437.0, 452.0, 340.0, 331.0, 325.0, 299.0, 239.0, 269.0, 231.0, 196.0, 210.0, 170.0, 223.0, 212.0, 190.0, 193.0, 208.0, 191.0, 194.0, 208.0, 190.0, 199.0, 189.0, 169.0, 162.0, 174.0, 152.0, 150.0, 186.0, 155.0, 175.0, 197.0, 186.0, 190.0, 193.0, 168.0, 171.0, 195.0, 176.0, 177.0, 161.0, 155.0, 152.0, 150.0, 172.0, 157.0, 187.0, 164.0, 159.0, 177.0, 191.0, 164.0, 175.0, 176.0, 154.0, 160.0, 150.0, 165.0, 160.0, 147.0, 158.0, 141.0, 166.0, 171.0, 147.0, 152.0, 183.0, 171.0, 189.0, 142.0, 152.0, 159.0, 134.0, 168.0, 168.0, 145.0, 164.0, 149.0, 161.0, 176.0, 161.0, 189.0, 168.0, 170.0, 170.0, 171.0, 182.0, 170.0, 150.0, 179.0, 182.0, 169.0, 156.0, 165.0, 160.0, 177.0, 141.0, 159.0, 171.0, 170.0, 160.0, 181.0, 171.0, 157.0, 151.0, 169.0, 161.0, 151.0, 185.0, 152.0, 150.0, 153.0, 159.0, 187.0, 174.0, 173.0, 148.0, 176.0, 186.0, 166.0, 152.0, 155.0, 148.0, 141.0, 159.0, 165.0, 139.0, 144.0, 165.0, 165.0, 161.0, 163.0, 182.0, 162.0, 138.0, 179.0, 178.0, 164.0, 167.0, 173.0, 167.0, 175.0, 156.0, 159.0, 156.0, 148.0, 189.0, 161.0, 151.0, 165.0, 153.0, 166.0, 157.0, 164.0, 165.0, 153.0, 169.0, 167.0, 167.0, 146.0, 163.0, 162.0, 170.0, 171.0, 180.0, 188.0, 164.0, 180.0, 156.0, 149.0, 170.0, 153.0, 160.0, 164.0, 158.0, 160.0, 156.0, 159.0, 165.0, 146.0, 142.0, 136.0, 178.0, 159.0, 155.0, 176.0, 181.0, 156.0, 173.0, 169.0, 158.0, 181.0, 162.0, 164.0, 168.0, 160.0, 173.0, 164.0, 170.0, 179.0, 170.0, 145.0, 160.0, 162.0, 138.0, 153.0, 179.0, 154.0, 181.0, 178.0, 173.0, 180.0, 172.0, 168.0, 179.0, 163.0, 158.0, 150.0, 141.0, 135.0, 170.0, 156.0, 142.0, 148.0, 154.0, 152.0, 170.0, 144.0, 172.0, 152.0, 164.0, 156.0, 160.0, 141.0, 149.0, 155.0, 148.0, 181.0, 168.0, 175.0, 169.0, 166.0, 172.0, 167.0, 187.0, 152.0, 156.0, 178.0, 175.0, 160.0, 175.0]
  out "Off-Line Smoothed":dbl[](array[numeric])=[500.25531914893617, 753.7340425531913, 986.7287234042552, 1160.4521276595742, 1267.2446808510635, 1303.6595744680847, 1285.5212765957442, 1233.696808510638, 1156.4521276595742, 1071.1702127659573, 989.7765957446807, 914.3297872340424, 847.3989361702127, 788.1117021276593, 732.7765957446808, 676.8031914893617, 626.5372340425531, 583.031914893617, 540.8404255319149, 502.73404255319144, 471.8936170212766, 442.436170212766, 411.3936170212766, 386.17553191489367, 358.89893617021283, 327.38829787234056, 302.60638297872345, 280.27127659574467, 254.54787234042556, 220.5053191489362, 180.16489361702128, 146.96276595744683, 123.70212765957446, 104.89893617021275, 91.2446808510638, 83.54255319148933, 74.25531914893617, 67.88829787234042, 63.196808510638284, 57.69680851063829, 55.34042553191489, 49.617021276595736, 44.75, 41.037234042553195, 37.04255319148936, 33.87765957446808, 31.643617021276597, 28.95744680851064, 26.941489361702132, 26.308510638297875, 23.962765957446813, 23.17021276595745, 20.88829787234043, 17.010638297872347, 16.361702127659584, 15.047872340425538, 12.547872340425533, 13.468085106382981, 15.313829787234047, 15.521276595744684, 14.930851063829792, 12.308510638297873, 11.297872340425531, 10.78191489361702, 8.936170212765953, 7.787234042553187, 7.159574468085102, 7.276595744680846, 5.617021276595743, 4.601063829787234, 6.30851063829787, 6.819148936170209, 5.867021276595741, 6.1170212765957395, 6.739361702127654, 5.382978723404253, 3.8031914893617023, 4.340425531914893, 5.0478723404255295, 4.7234042553191475, 4.404255319148935, 4.324468085106381, 3.1861702127659566, 2.6914893617021276, 3.8936170212765955, 3.2180851063829787, 3.53191489361702, 4.191489361702127, 3.0319148936170213, 3.1117021276595747, 3.4787234042553186, 3.2712765957446805, 3.3404255319148937, 3.808510638297871, 4.882978723404253, 3.984042553191489, 2.632978723404255, 1.877659574468085, 1.7340425531914894, 3.292553191489362, 3.5, 3.5478723404255303, 2.909574468085105, 2.175531914893617, 2.2074468085106385, 2.686170212765957, 2.5797872340425525, 1.6170212765957448, 1.9574468085106382, 2.7712765957446805, 2.6861702127659575, 2.6968085106382977, 2.904255319148936, 2.622340425531915, 1.5691489361702127, 1.4574468085106382, 2.1914893617021276, 3.117021276595744, 3.446808510638297, 1.5797872340425532, 0.1648936170212766, 0.8617021276595745, 0.9148936170212767, 0.23404255319148937, 0.5319148936170213, -0.23404255319148937, -0.4734042553191489, 1.9946808510638299, 4.542553191489361, 2.654255319148936, 0.4148936170212766, 0.5319148936170213, 0.6914893617021276, 1.297872340425532, 2.202127659574468, 1.3457446808510638, 0.2074468085106383, -0.40957446808510634, 0.7819148936170214, 2.8031914893617023, 2.1968085106382977, 1.0425531914893618, 0.0, 0.23404255319148937, 1.2180851063829787, 0.8404255319148936, 0.0797872340425532, -0.06914893617021275, 0.9734042553191489, 1.9042553191489362, 0.6117021276595744, 0.5904255319148937, 1.5106382978723405, 1.6755319148936172, 0.973404255319149, -0.06382978723404255, 1.3191489361702127, 1.9361702127659575, 0.7872340425531915, 1.5319148936170208, 2.457446808510638, -0.2340425531914896, -2.1010638297872344, -0.30319148936170215, 0.7287234042553192, 0.6382978723404256, 0.5957446808510638, 0.6170212765957447, 1.9202127659574462, 1.4255319148936163, 1.8351063829787233, 1.3031914893617023, -0.03191489361702127, 0.2819148936170212, 1.276595744680851, 1.7606382978723403, -0.6808510638297872, -0.7340425531914894, 1.2074468085106382, 1.0851063829787233, 0.4627659574468085, -0.5319148936170214, -0.574468085106383, 1.047872340425532, 2.4680851063829787, 2.404255319148936, 0.6329787234042553, 0.13829787234042554, -0.03191489361702128, -0.8617021276595744, -1.702127659574468, -1.3617021276595744, -1.0, -1.7393617021276595, -1.4840425531914894, -0.8351063829787233, -0.9308510638297872, -0.22872340425531915, -0.6063829787234042, 0.02659574468085113, 1.5797872340425534, 1.271276595744681, 1.6117021276595744, 0.5159574468085106, -1.6648936170212767, -0.7127659574468086, 1.2553191489361701, 0.5425531914893618, 0.6968085106382977, 1.9468085106382977, 2.5425531914893615, 1.5691489361702127, -0.6063829787234043, 1.0106382978723392, 2.659574468085105, 1.058510638297872, 1.4734042553191489, 2.25531914893617, 0.5797872340425532, -0.5478723404255319, -0.10638297872340424, 0.5957446808510638, -0.6436170212765957, -0.22872340425531912, 1.122340425531915, 0.7393617021276595, -0.20744680851063835, -0.7712765957446809, 1.452127659574468, 1.5585106382978724, -0.22872340425531915, -0.2393617021276596, 0.7127659574468085, 0.8936170212765957, 0.7021276595744681, 0.6595744680851064, 0.39893617021276595, 0.8617021276595744, 0.7872340425531915, -0.10638297872340424, -0.7765957446808511, 0.5319148936170213, 0.010638297872340385, -0.6117021276595745, 0.2978723404255319, 0.02127659574468084, 0.2978723404255319, -0.03723404255319146, -0.17553191489361702, 0.5, 0.3617021276595745, 0.48936170212765956, 0.601063829787234, 0.6276595744680851, 0.7606382978723404, 0.11170212765957444, -0.8776595744680851, -0.6382978723404255, 0.5691489361702128, 0.48936170212765956, -0.7393617021276595, -0.18085106382978722, 1.4308510638297873, 0.08510638297872342, -0.7606382978723404, -0.16489361702127658, 0.32446808510638303, 0.3297872340425532, -0.38829787234042556, -0.7340425531914894, -0.9627659574468086, -0.30851063829787234, -0.10106382978723404, -0.5053191489361701, 0.08510638297872342, 1.521276595744681, 1.5904255319148937]
  out "On-Line  Smoothed":dbl[](array[numeric])=[597.5521276595745, 853.2223404255317, 1061.5521276595741, 1186.7968085106381, 1234.8393617021275, 1216.7382978723401, 1147.6744680851061, 1056.7542553191486, 955.8712765957443, 854.5840425531912, 757.887234042553, 671.0946808510637, 597.8393617021275, 534.0999999999999, 478.23297872340424, 425.163829787234, 379.12127659574463, 343.0095744680852, 310.2170212765958, 277.23297872340436, 248.02021276595752, 224.76489361702136, 207.1478723404256, 188.7329787234043, 165.88723404255322, 144.44574468085108, 130.0468085106383, 118.68510638297872, 104.39255319148936, 88.76489361702127, 71.27021276595742, 56.280851063829765, 48.06276595744679, 41.20106382978722, 34.732978723404244, 30.19042553191489, 27.32872340425532, 24.998936170212765, 22.61063829787234, 19.70638297872341, 17.96702127659575, 16.472340425531918, 14.929787234042555, 14.211702127659574, 13.211702127659574, 12.435106382978724, 11.206382978723406, 10.254255319148937, 10.59468085106383, 8.982978723404255, 6.722340425531915, 6.004255319148935, 5.169148936170211, 5.254255319148937, 4.610638297872341, 4.2968085106382965, 3.8978723404255318, 3.5946808510638304, 3.068085106382979, 1.3712765957446813, 2.408510638297872, 3.578723404255319, 4.482978723404255, 4.179787234042552, 2.828723404255319, 2.3659574468085105, 1.6425531914893616, 1.3180851063829786, 0.3712765957446811, 0.4936170212765958, 0.9829787234042553, 2.3712765957446806, 2.8978723404255313, 2.732978723404255, 2.073404255319149, 1.7436170212765958, 1.2968085106382978, 2.020212765957447, 2.4829787234042553, -0.10744680851063809, 1.3553191489361702, 2.296808510638298, 1.7702127659574467, 2.121276595744681, 0.5414893617021278, 0.7223404255319149, 1.3074468085106383, 1.1212765957446806, 1.0095744680851062, 0.33404255319148957, 0.17446808510638318, 0.020212765957447032, 1.2808510638297872, 1.9191489361702128, 1.0042553191489363, 1.424468085106383, 0.9510638297872341, 1.3180851063829788, 1.3872340425531915, 0.9457446808510639, 1.3393617021276596, -0.03829787234042534, 0.19574468085106406, 1.35531914893617, 2.482978723404255, 1.8553191489361702, -0.431914893617021, 0.6159574468085104, 1.057446808510638, 0.5361702127659573, 1.6957446808510632, 1.0255319148936168, 0.1319148936170215, 1.1638297872340426, 3.0414893617021272, 2.2542553191489363, 1.5840425531914895, 1.2436170212765958, 0.10000000000000021, -0.9851063829787235, -1.2031914893617024, -0.38936170212765936, 0.11063829787234061, 0.9936170212765958, 1.9031914893617021, 1.4829787234042557, -0.7989361702127658, -1.5968085106382977, -1.3414893617021275, 0.1797872340425526, 0.1904255319148931, -0.13936170212765975, -0.06489361702127683, -1.2776595744680854, -1.421276595744681, -0.4265957446808512, 1.3287234042553187, 0.9191489361702125, 0.21170212765957466, -0.0010638297872338498, -0.5968085106382977, -0.6180851063829785, -0.2882978723404253, 0.5148936170212768, 0.6904255319148939, 1.3819148936170211, 2.0787234042553187, 0.5042553191489363, -0.7244680851063825, -0.1925531914893615, 0.29680851063829805, -0.04361702127659553, 0.8978723404255322, 0.8021276595744682, 1.2010638297872338, 2.5042553191489354, 1.0946808510638295, 0.6744680851063831, 1.9617021276595745, 0.9191489361702129, 0.2648936170212768, 2.541489361702127, 2.823404255319148, 1.738297872340425, 0.49361702127659557, -0.5595744680851062, 0.15851063829787254, 0.2170212765957448, 1.451063829787234, 2.514893617021276, 0.9882978723404254, -0.29893617021276575, -0.09680851063829765, 0.770212765957447, 0.11063829787234064, 0.08404255319148957, 0.5308510638297874, 0.3287234042553194, 0.8553191489361704, 0.2755319148936173, -0.5436170212765955, -0.8787234042553193, -1.6872340425531922, -1.2776595744680854, -0.5542553191489359, 0.4085106382978725, 1.1425531914893619, 0.47234042553191513, -1.1606382978723402, -0.8680851063829784, -0.22978723404255313, -0.926595744680851, -1.3361702127659574, -1.1872340425531913, 0.3659574468085106, 1.1053191489361707, 0.5202127659574474, 0.3925531914893619, 1.2808510638297874, 0.6319148936170214, 0.6744680851063831, 1.5946808510638302, 1.1957446808510643, 0.38191489361702147, -0.4425531914893615, -0.9904255319148938, -1.1074468085106386, 0.07340425531914907, -0.14999999999999986, -0.4425531914893615, 0.796808510638298, 2.0095744680851064, 1.6957446808510637, 0.009574468085106591, -0.1925531914893615, -0.29361702127659556, 1.2223404255319148, 2.7702127659574463, 0.39787234042553155, -0.6765957446808509, -0.12340425531914874, 0.3712765957446812, -0.38936170212765964, -0.8414893617021278, -0.20319148936170195, -0.4106382978723404, 0.35000000000000003, 0.8021276595744683, 0.31808510638297893, 0.3287234042553196, 1.2382978723404257, 1.2010638297872338, -0.39999999999999997, -1.0010638297872338, -0.1925531914893615, 0.036170212765957666, -0.44255319148936145, -0.4212765957446806, 0.802127659574468, 0.12659574468085055, -0.01170212765957468, 1.5202127659574467, 1.2861702127659573, 1.0946808510638302, 1.0255319148936175, 0.5095744680851066, -0.1606382978723402, 0.4404255319148939, 0.6212765957446812, -1.14468085106383, -1.7404255319148936, -0.6712765957446806, 0.3765957446808513, 0.9457446808510641, 0.892553191489362, 0.33404255319148957, -0.22978723404255322, 0.3021276595744678, 0.5468085106382978, -0.4531914893617019, -0.18191489361702096, 0.6531914893617023, 0.13191489361702147, -0.6765957446808508, -0.04893617021276575, 0.7117021276595747, 0.5148936170212768, 0.39255319148936185, -0.42127659574468074, -0.777659574468085, -0.2404255319148934, 0.24361702127659599, 0.14787234042553216, -0.330851063829787, 0.10531914893617042, 0.8287234042553194, 0.37127659574468114]
  out "On-Line Bin Readings":dbl[](array[numeric])=[603.0, 872.0, 1149.0, 1254.0, 1388.0, 1468.0, 1439.0, 1303.0, 1193.0, 1062.0, 935.0, 860.0, 840.0, 680.0, 636.0, 611.0, 547.0, 484.0, 463.0, 427.0, 381.0, 353.0, 314.0, 321.0, 285.0, 305.0, 283.0, 261.0, 245.0, 225.0, 201.0, 186.0, 200.0, 164.0, 173.0, 150.0, 162.0, 158.0, 151.0, 164.0, 162.0, 143.0, 134.0, 124.0, 118.0, 145.0, 132.0, 129.0, 135.0, 140.0, 104.0, 117.0, 126.0, 118.0, 127.0, 132.0, 140.0, 138.0, 141.0, 120.0, 120.0, 131.0, 130.0, 153.0, 122.0, 117.0, 146.0, 133.0, 119.0, 131.0, 130.0, 127.0, 122.0, 118.0, 110.0, 144.0, 141.0, 119.0, 136.0, 115.0, 132.0, 144.0, 116.0, 137.0, 138.0, 104.0, 117.0, 114.0, 130.0, 124.0, 151.0, 119.0, 117.0, 136.0, 140.0, 102.0, 122.0, 120.0, 121.0, 125.0, 134.0, 113.0, 138.0, 160.0, 106.0, 125.0, 136.0, 120.0, 122.0, 129.0, 131.0, 130.0, 111.0, 115.0, 114.0, 118.0, 118.0, 125.0, 135.0, 124.0, 127.0, 139.0, 144.0, 126.0, 118.0, 140.0, 131.0, 115.0, 123.0, 137.0, 129.0, 137.0, 108.0, 137.0, 107.0, 106.0, 114.0, 117.0, 93.0, 139.0, 137.0, 106.0, 104.0, 136.0, 116.0, 128.0, 123.0, 139.0, 114.0, 109.0, 132.0, 113.0, 122.0, 125.0, 112.0, 116.0, 119.0, 126.0, 140.0, 113.0, 107.0, 115.0, 139.0, 126.0, 99.0, 108.0, 116.0, 132.0, 118.0, 143.0, 118.0, 139.0, 124.0, 120.0, 127.0, 119.0, 128.0, 112.0, 143.0, 154.0, 143.0, 130.0, 147.0, 124.0, 126.0, 112.0, 111.0, 111.0, 109.0, 149.0, 105.0, 121.0, 135.0, 123.0, 107.0, 121.0, 130.0, 127.0, 148.0, 113.0, 131.0, 116.0, 133.0, 136.0, 146.0, 111.0, 118.0, 120.0, 147.0, 129.0, 117.0, 140.0, 126.0, 120.0, 129.0, 119.0, 125.0, 123.0, 146.0, 109.0, 141.0, 102.0, 143.0, 112.0, 121.0, 134.0, 135.0, 109.0, 121.0, 125.0, 131.0, 112.0, 120.0, 116.0, 116.0, 119.0, 129.0, 119.0, 140.0, 116.0, 137.0, 130.0, 127.0, 116.0, 127.0, 137.0, 141.0, 123.0, 136.0, 138.0, 126.0, 108.0, 125.0, 127.0, 129.0, 110.0, 110.0, 120.0, 111.0, 114.0, 127.0, 108.0, 142.0, 132.0, 108.0, 110.0, 126.0, 106.0, 132.0, 125.0, 131.0, 120.0, 124.0, 120.0, 116.0, 109.0, 124.0, 116.0, 134.0]
  out "Range Corrected Altitude Array":dbl[](array[numeric])=[5625.0, 22500.0, 50625.0, 90000.0, 140625.0, 202500.0, 275625.0, 360000.0, 455625.0, 562500.0, 680625.0, 810000.0, 950625.0, 1102500.0, 1265625.0, 1440000.0, 1625625.0, 1822500.0, 2030625.0, 2250000.0, 2480625.0, 2722500.0, 2975625.0, 3240000.0, 3515625.0, 3802500.0, 4100625.0, 4410000.0, 4730625.0, 5062500.0, 5405625.0, 5760000.0, 6125625.0, 6502500.0, 6890625.0, 7290000.0, 7700625.0, 8122500.0, 8555625.0, 9000000.0, 9455625.0, 9922500.0, 10400625.0, 10890000.0, 11390625.0, 11902500.0, 12425625.0, 12960000.0, 13505625.0, 14062500.0, 14630625.0, 15210000.0, 15800625.0, 16402500.0, 17015625.0, 17640000.0, 18275625.0, 18922500.0, 19580625.0, 20250000.0, 20930625.0, 21622500.0, 22325625.0, 23040000.0, 23765625.0, 24502500.0, 25250625.0, 26010000.0, 26780625.0, 27562500.0, 28355625.0, 29160000.0, 29975625.0, 30802500.0, 31640625.0, 32490000.0, 33350625.0, 34222500.0, 35105625.0, 36000000.0, 36905625.0, 37822500.0, 38750625.0, 39690000.0, 40640625.0, 41602500.0, 42575625.0, 43560000.0, 44555625.0, 45562500.0, 46580625.0, 47610000.0, 48650625.0, 49702500.0, 50765625.0, 51840000.0, 52925625.0, 54022500.0, 55130625.0, 56250000.0, 57380625.0, 58522500.0, 59675625.0, 60840000.0, 62015625.0, 63202500.0, 64400625.0, 65610000.0, 66830625.0, 68062500.0, 69305625.0, 70560000.0, 71825625.0, 73102500.0, 74390625.0, 75690000.0, 77000625.0, 78322500.0, 79655625.0, 81000000.0, 82355625.0, 83722500.0, 85100625.0, 86490000.0, 87890625.0, 89302500.0, 90725625.0, 92160000.0, 93605625.0, 95062500.0, 96530625.0, 98010000.0, 99500625.0, 101002500.0, 102515625.0, 104040000.0, 105575625.0, 107122500.0, 108680625.0, 110250000.0, 111830625.0, 113422500.0, 115025625.0, 116640000.0, 118265625.0, 119902500.0, 121550625.0, 123210000.0, 124880625.0, 126562500.0, 128255625.0, 129960000.0, 131675625.0, 133402500.0, 135140625.0, 136890000.0, 138650625.0, 140422500.0, 142205625.0, 144000000.0, 145805625.0, 147622500.0, 149450625.0, 151290000.0, 153140625.0, 155002500.0, 156875625.0, 158760000.0, 160655625.0, 162562500.0, 164480625.0, 166410000.0, 168350625.0, 170302500.0, 172265625.0, 174240000.0, 176225625.0, 178222500.0, 180230625.0, 182250000.0, 184280625.0, 186322500.0, 188375625.0, 190440000.0, 192515625.0, 194602500.0, 196700625.0, 198810000.0, 200930625.0, 203062500.0, 205205625.0, 207360000.0, 209525625.0, 211702500.0, 213890625.0, 216090000.0, 218300625.0, 220522500.0, 222755625.0, 225000000.0, 227255625.0, 229522500.0, 231800625.0, 234090000.0, 236390625.0, 238702500.0, 241025625.0, 243360000.0, 245705625.0, 248062500.0, 250430625.0, 252810000.0, 255200625.0, 257602500.0, 260015625.0, 262440000.0, 264875625.0, 267322500.0, 269780625.0, 272250000.0, 274730625.0, 277222500.0, 279725625.0, 282240000.0, 284765625.0, 287302500.0, 289850625.0, 292410000.0, 294980625.0, 297562500.0, 300155625.0, 302760000.0, 305375625.0, 308002500.0, 310640625.0, 313290000.0, 315950625.0, 318622500.0, 321305625.0, 324000000.0, 326705625.0, 329422500.0, 332150625.0, 334890000.0, 337640625.0, 340402500.0, 343175625.0, 345960000.0, 348755625.0, 351562500.0, 354380625.0, 357210000.0, 360050625.0, 362902500.0, 365765625.0, 368640000.0, 371525625.0, 374422500.0, 377330625.0, 380250000.0, 383180625.0, 386122500.0, 389075625.0, 392040000.0, 395015625.0, 398002500.0, 401000625.0, 404010000.0, 407030625.0, 410062500.0, 413105625.0, 416160000.0, 419225625.0, 422302500.0, 425390625.0, 428490000.0, 431600625.0, 434722500.0, 437855625.0, 441000000.0]
  out "Altitude Array (km)":dbl[](array[numeric])=[0.075, 0.15, 0.22499999999999998, 0.3, 0.375, 0.45, 0.5249999999999999, 0.6, 0.6749999999999999, 0.7499999999999999, 0.825, 0.8999999999999999, 0.9749999999999999, 1.05, 1.125, 1.2, 1.275, 1.3499999999999999, 1.4249999999999998, 1.5, 1.575, 1.65, 1.7249999999999999, 1.7999999999999998, 1.8749999999999998, 1.95, 2.025, 2.1, 2.1750000000000003, 2.25, 2.325, 2.4, 2.475, 2.5500000000000003, 2.625, 2.7, 2.775, 2.85, 2.9250000000000003, 3.0, 3.075, 3.15, 3.225, 3.3000000000000003, 3.375, 3.45, 3.525, 3.6, 3.675, 3.75, 3.825, 3.9, 3.975, 4.05, 4.125, 4.2, 4.275, 4.35, 4.425, 4.5, 4.575, 4.65, 4.725, 4.8, 4.875, 4.95, 5.025, 5.1, 5.175, 5.25, 5.325, 5.4, 5.475, 5.55, 5.625, 5.7, 5.775, 5.85, 5.925, 6.0, 6.075, 6.15, 6.225, 6.3, 6.375, 6.45, 6.525, 6.6, 6.675, 6.75, 6.825, 6.9, 6.975, 7.05, 7.125, 7.2, 7.2749999999999995, 7.35, 7.425, 7.5, 7.575, 7.6499999999999995, 7.725, 7.8, 7.875, 7.95, 8.024999999999999, 8.1, 8.174999999999999, 8.249999999999998, 8.325, 8.399999999999999, 8.475, 8.549999999999999, 8.624999999999998, 8.7, 8.774999999999999, 8.85, 8.924999999999999, 8.999999999999998, 9.075, 9.149999999999999, 9.225, 9.299999999999999, 9.374999999999998, 9.45, 9.524999999999999, 9.6, 9.674999999999999, 9.749999999999998, 9.825, 9.899999999999999, 9.975, 10.049999999999999, 10.124999999999998, 10.2, 10.274999999999999, 10.35, 10.424999999999999, 10.499999999999998, 10.575, 10.649999999999999, 10.725, 10.799999999999999, 10.874999999999998, 10.95, 11.024999999999999, 11.1, 11.174999999999999, 11.249999999999998, 11.325, 11.399999999999999, 11.475, 11.549999999999999, 11.624999999999998, 11.7, 11.774999999999999, 11.85, 11.924999999999999, 11.999999999999998, 12.075, 12.149999999999999, 12.225, 12.299999999999999, 12.374999999999998, 12.45, 12.524999999999999, 12.6, 12.674999999999999, 12.749999999999998, 12.825, 12.899999999999999, 12.975, 13.049999999999999, 13.124999999999998, 13.2, 13.274999999999999, 13.35, 13.424999999999999, 13.499999999999998, 13.575, 13.649999999999999, 13.725, 13.799999999999999, 13.874999999999998, 13.95, 14.024999999999999, 14.1, 14.174999999999999, 14.249999999999998, 14.325, 14.399999999999999, 14.474999999999998, 14.549999999999999, 14.624999999999998, 14.7, 14.774999999999999, 14.849999999999998, 14.924999999999999, 14.999999999999998, 15.075, 15.149999999999999, 15.224999999999998, 15.299999999999999, 15.374999999999998, 15.45, 15.524999999999999, 15.599999999999998, 15.674999999999999, 15.749999999999998, 15.825, 15.899999999999999, 15.974999999999998, 16.05, 16.125, 16.2, 16.275, 16.349999999999998, 16.424999999999997, 16.5, 16.575, 16.65, 16.724999999999998, 16.799999999999997, 16.875, 16.95, 17.025, 17.099999999999998, 17.174999999999997, 17.25, 17.325, 17.4, 17.474999999999998, 17.549999999999997, 17.625, 17.7, 17.775, 17.849999999999998, 17.924999999999997, 18.0, 18.075, 18.15, 18.224999999999998, 18.299999999999997, 18.375, 18.45, 18.525, 18.599999999999998, 18.674999999999997, 18.75, 18.825, 18.9, 18.974999999999998, 19.049999999999997, 19.125, 19.2, 19.275, 19.349999999999998, 19.424999999999997, 19.5, 19.575, 19.65, 19.724999999999998, 19.799999999999997, 19.875, 19.95, 20.025, 20.099999999999998, 20.174999999999997, 20.25, 20.325, 20.4, 20.474999999999998, 20.549999999999997, 20.625, 20.7, 20.775, 20.849999999999998, 20.924999999999997, 21.0]
  out "Offline Pulse Energy":dbl=3.240295714285714
  out "Online Pulse Energy":dbl=3.2240871428571425
  in  "Instrument Control":T5(tab)=enum."Wavemeter"
  in  "ILX Address On":dbl=1.0 min=0.0 step=1.0
  in  "ILX Address Off":dbl=2.0 min=0.0 step=1.0
  in  "OnLineLD":dbl=169.7
  in  "OffLineLD":dbl=172.62
  in  "Pulse B Polarity":enum32{"Low", "High"}(ring)=enum."High"
  in  "Pulse A Delay(ns)":u32=1040 min=80 max=327600
  in  "Pulse B Delay(ns)":u32=170000 min=80 max=327600 step=1
  in  "Accumulation Delay(ns)":u32=10 min=10 max=1270 step=1
  in  "Sync Pulse Polarity":enum32{"Low", "High"}(ring)=enum."High"
  in  "Pulse A Polarity":enum32{"Low", "High"}(ring)=enum."High"
  in  "Number of Bins":u32=280 min=2 max=4095 step=1
  in  "Number of Accumulates":u32=10000 min=1 max=32767 step=1
  in  "Time Resolution Per Bin(ns)":u32=500 min=5 max=1063 step=1
  in  "Lambda On Set (nm)":dbl=828.198 format="%.5f"
  out "Lambda On Read (nm)":dbl=828.1980544852847 format="%.5f"
  out "Lambda Off Read (nm)":dbl=828.2976418470136 format="%.5f"
  in  "Lambda Off Set (nm)":dbl=828.29765 format="%#.5f"
  in  "Bristol In":i32=5
  out "Bristol Out":i32
  out "AB_DIF":dbl=5.448528474971681e-05 format="%#_15g"
  out "NONAB_DIF":dbl=-8.152986424647679e-06 format="%#_15g"
  out "Wavelength Lock Online":bool=TRUE
  out "Wavelength Lock Offline":bool=TRUE
  in  "calculate absorption cross sections":bool
  in  "Smoothing Range":dbl=150.0
  in  "Total DIAL Integration Time (Minutes)":i32=3
  in  "Data Reads (number of loops)":i32=1
  in  "Total Aerosol Integration Time (Minutes)":dbl=0.5
  in  "Scalar Wait Time":u32=500
  out "Smoothed Bins":dbl=2.0
  in  "NewportIn":string
  in  "logging":bool
  out "Newport Device Key":string="1918-R 15120"
  in  "SampleSize":i32=2
  out "NewportRef":refnum<k24>
  in  "Switch Comm Port":refnum<visa-resource-name>="COM3"
  out "FF_On_Ref":refnum<file>
  out "FF_On_Ptr":i64=1750320 format="%.2p"
  out "FF_Off_Ref":refnum<file>
  out "FF_Off_Ptr":i64=1745744 format="%.2p"
  out "NF_On_Ref":refnum<file>
  out "NF_On_Ptr":i64=1750320 format="%.2p"
  out "NF_Off_Ref":refnum<file>
  out "NF_Off_Ptr":i64=1745744 format="%.2p"
  out "DataOpen":bool=TRUE
  out "File Path_Far Field (out)":string="C:\\Users\\H2ODial\\Desktop\\SharedTeleWVData\\160812FF\\21"
  out "File Path_Near Field (out)":string="C:\\Users\\H2ODial\\Desktop\\SharedTeleWVData\\160812NF\\21"
  in  "Data File DIR (in)":string="C:\\Users\\H2ODial\\Desktop\\SharedTeleWVData\\"
  in  "bins":u32=280 min=2 max=4095 step=1
  out "y offset":u32=10
  in  "ns scale":u32=500
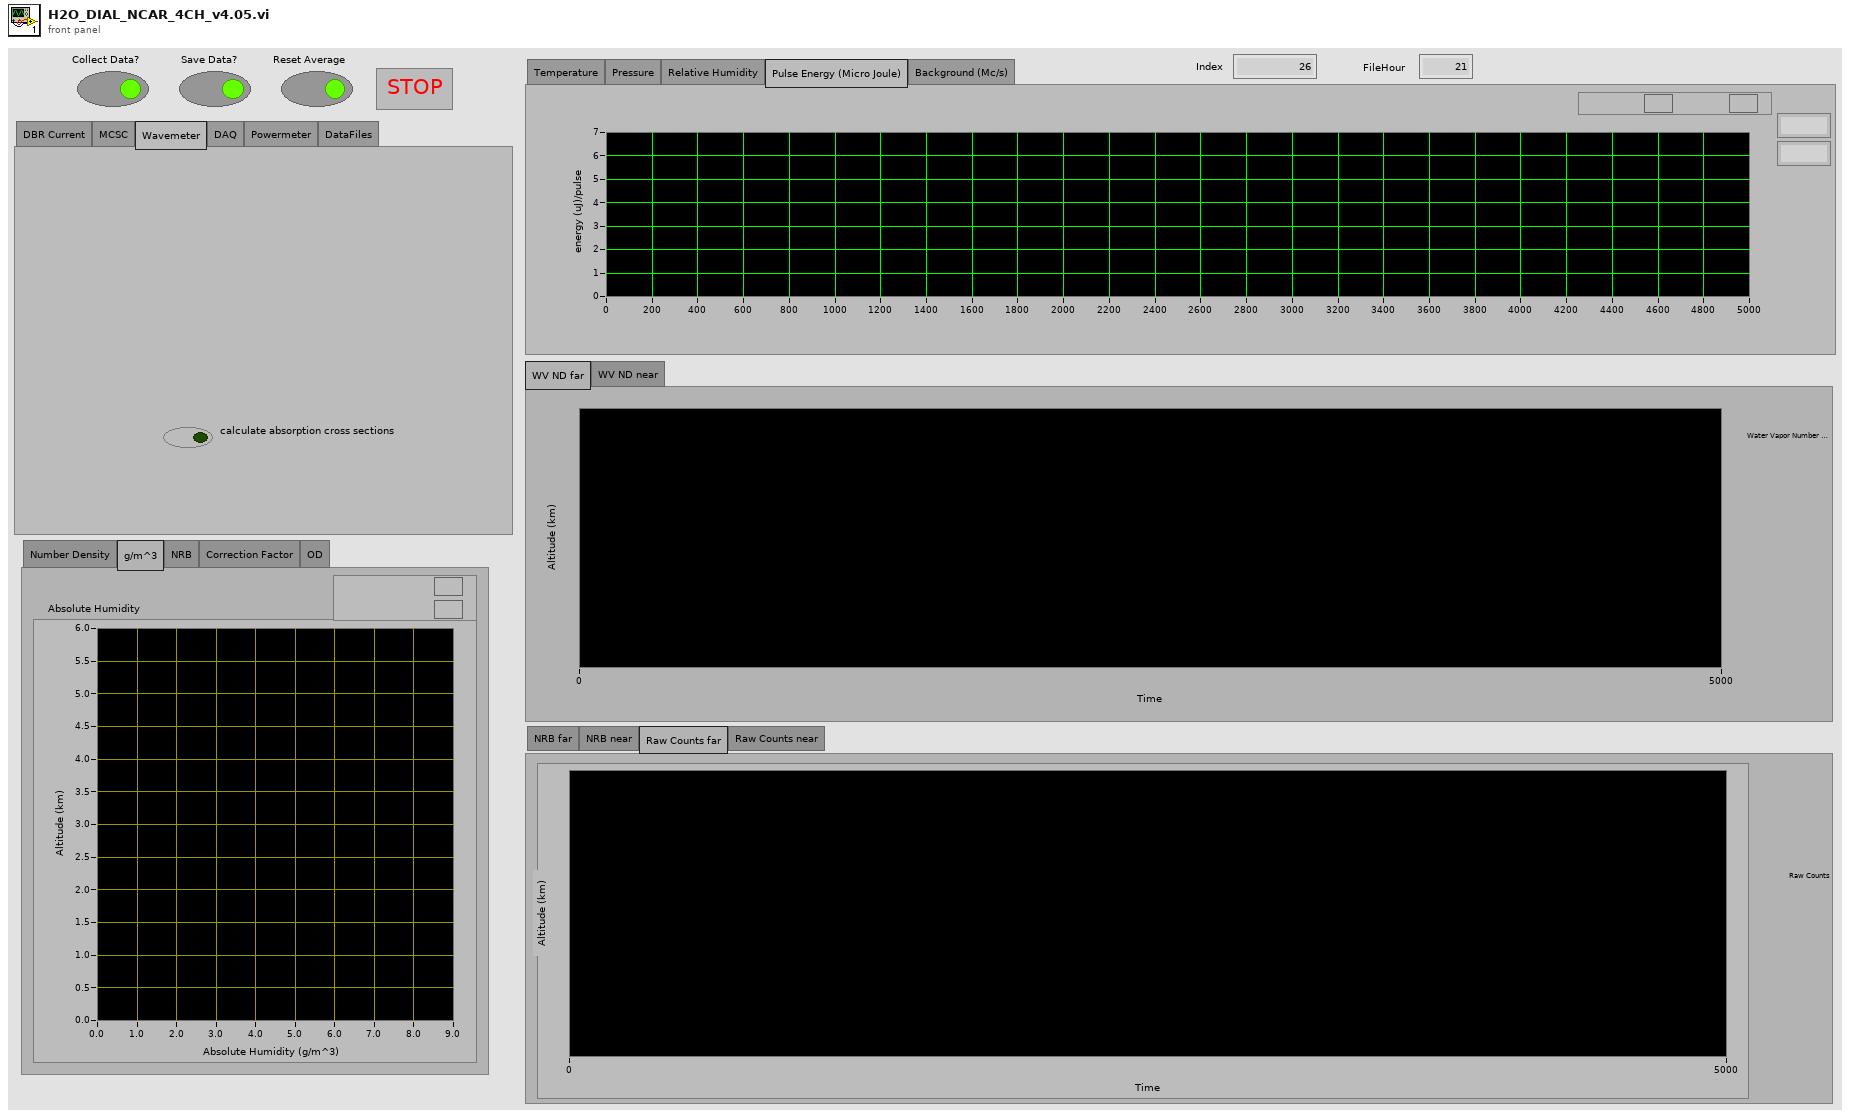
[diagram p1: front panel]
types:
  T1 = enum32{"NRB far", "NRB near", "Raw Counts far", "Raw Counts near"}
  T2 = enum32{"Number Density", "g/m^3", "NRB", "Correction Factor", "OD"}
  T3 = enum32{"Temperature", "Pressure", "Relative Humidity", "Pulse Energy (Micro Joule)", "Background (Mc/s)"}
  T4 = cluster{"Online Pulse Energy":dbl, "Pulse Energy Offline":dbl}
  T5 = enum32{"DBR Current", "MCSC", "Wavemeter", "DAQ", "Powermeter", "DataFiles"}
  T6 = enum16{"Initialize ILX", "Set ON T", "Set Off T", "Set ON I", "Set Off I", "Set On Lim", "Set Off Lim", "Read ILX", "TEC ON/OFF", "LASER ON/OFF", "Status?", "ILX OFF"}
  T7 = enum16{"open", "replace", "create", "open or create", "replace or create", "replace or create with confirmation"}
  T8 = typedef "LVDateTimeRec.ctl" = cluster{"fractional second":dbl, "second":i32, "minute":i32, "hour":i32, "day of month":i32, "month":i32, "year":i32, "day of week":i32, "day of year":i32, "DST":i32}
  T9 = cluster{"Online Pulse Energy":dbl, "Offline Pulse Energy":dbl}
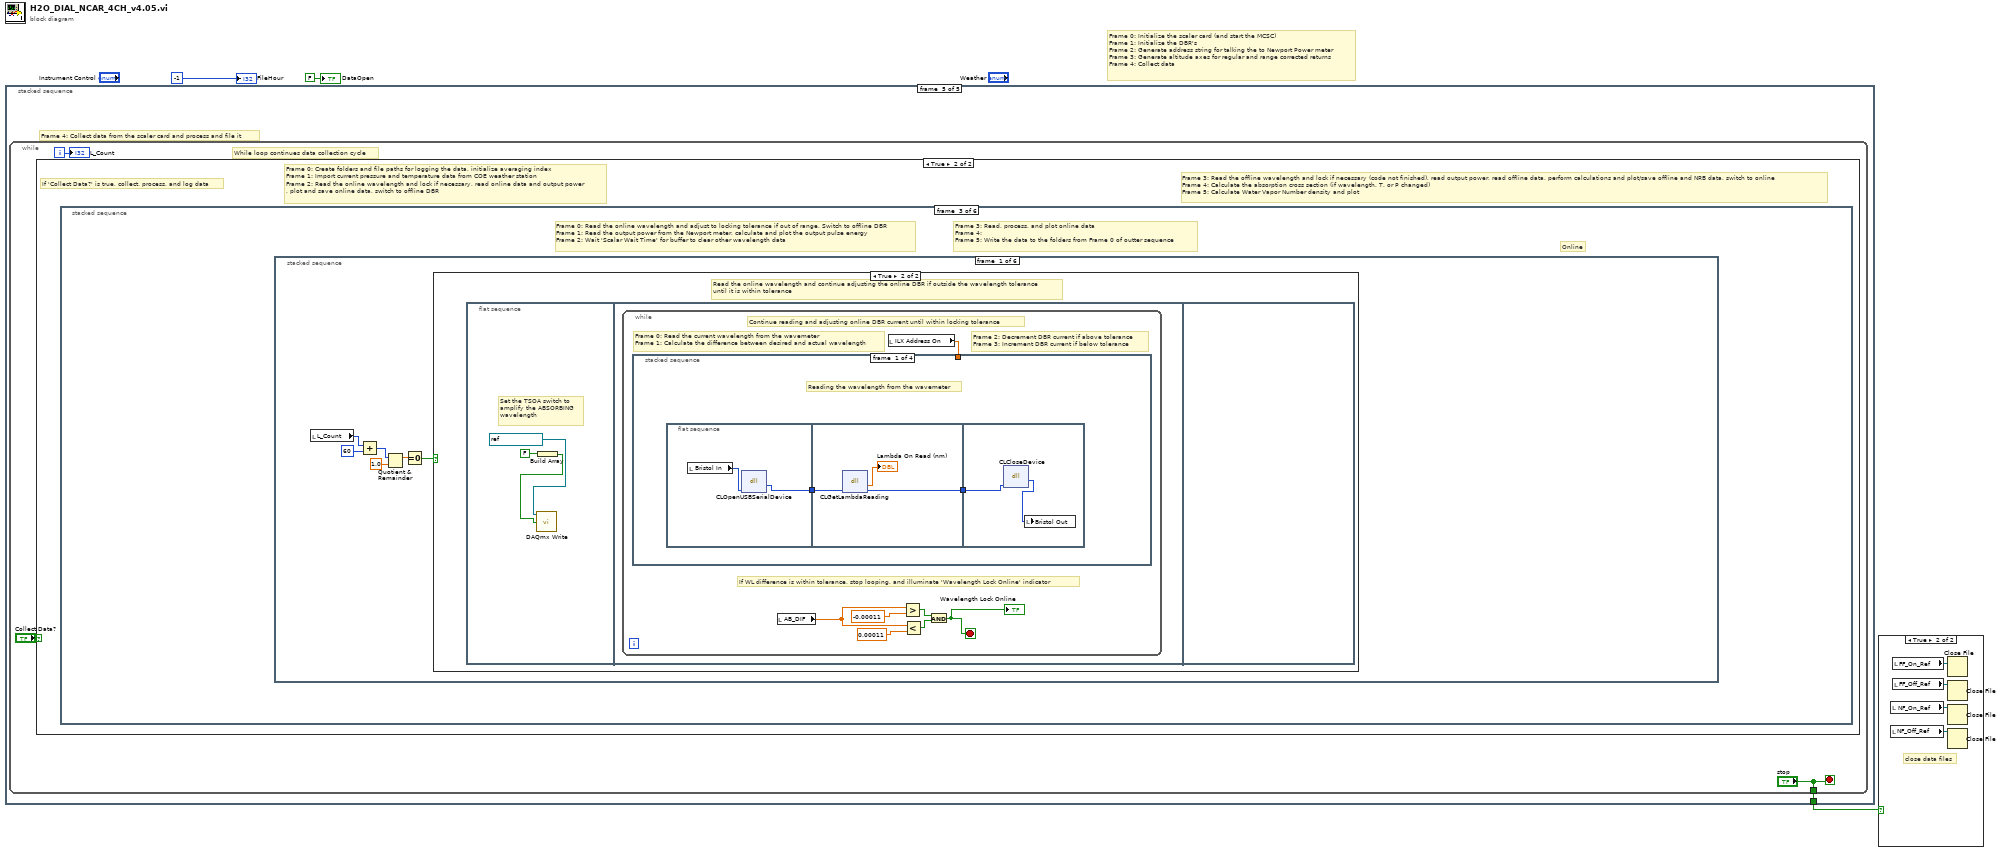
[diagram p0: block diagram]
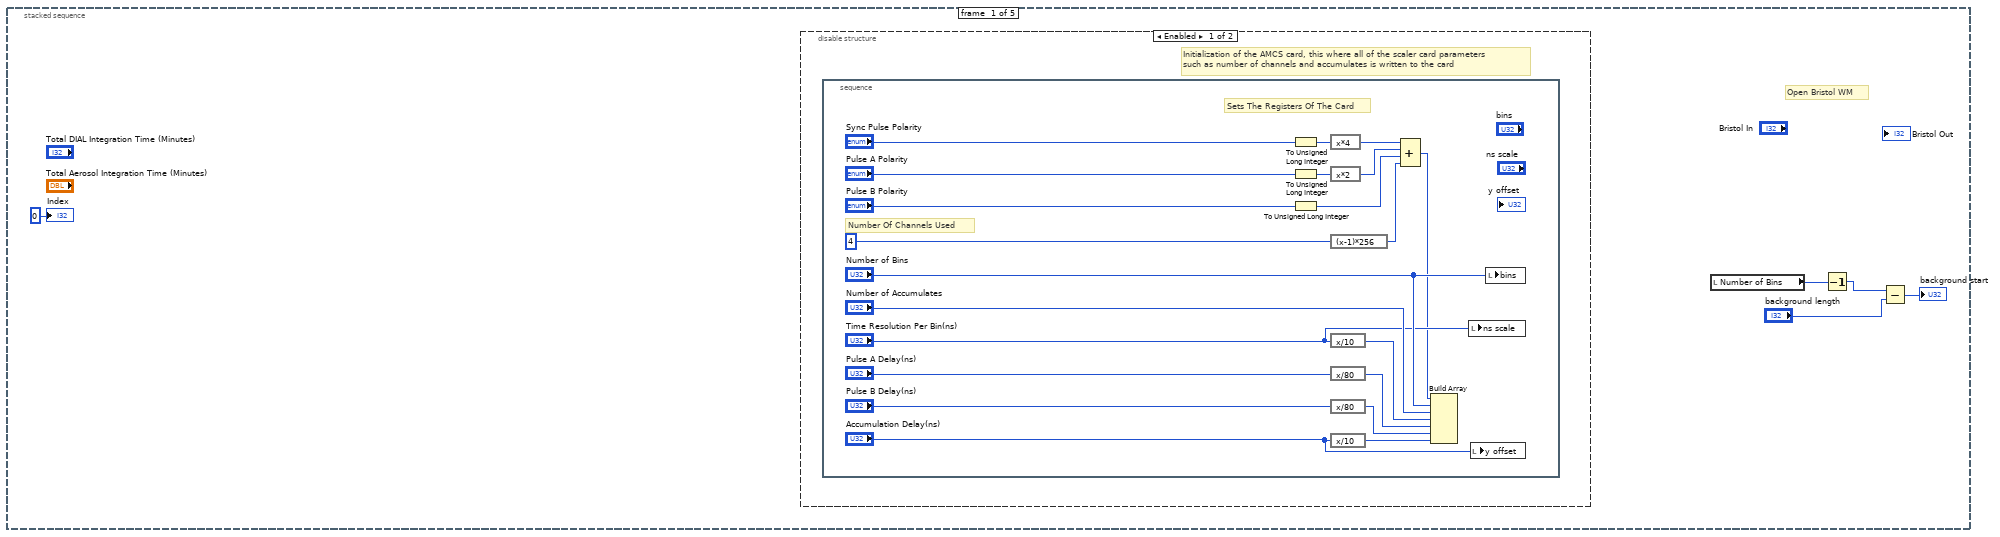
[diagram p3: hidden frame]
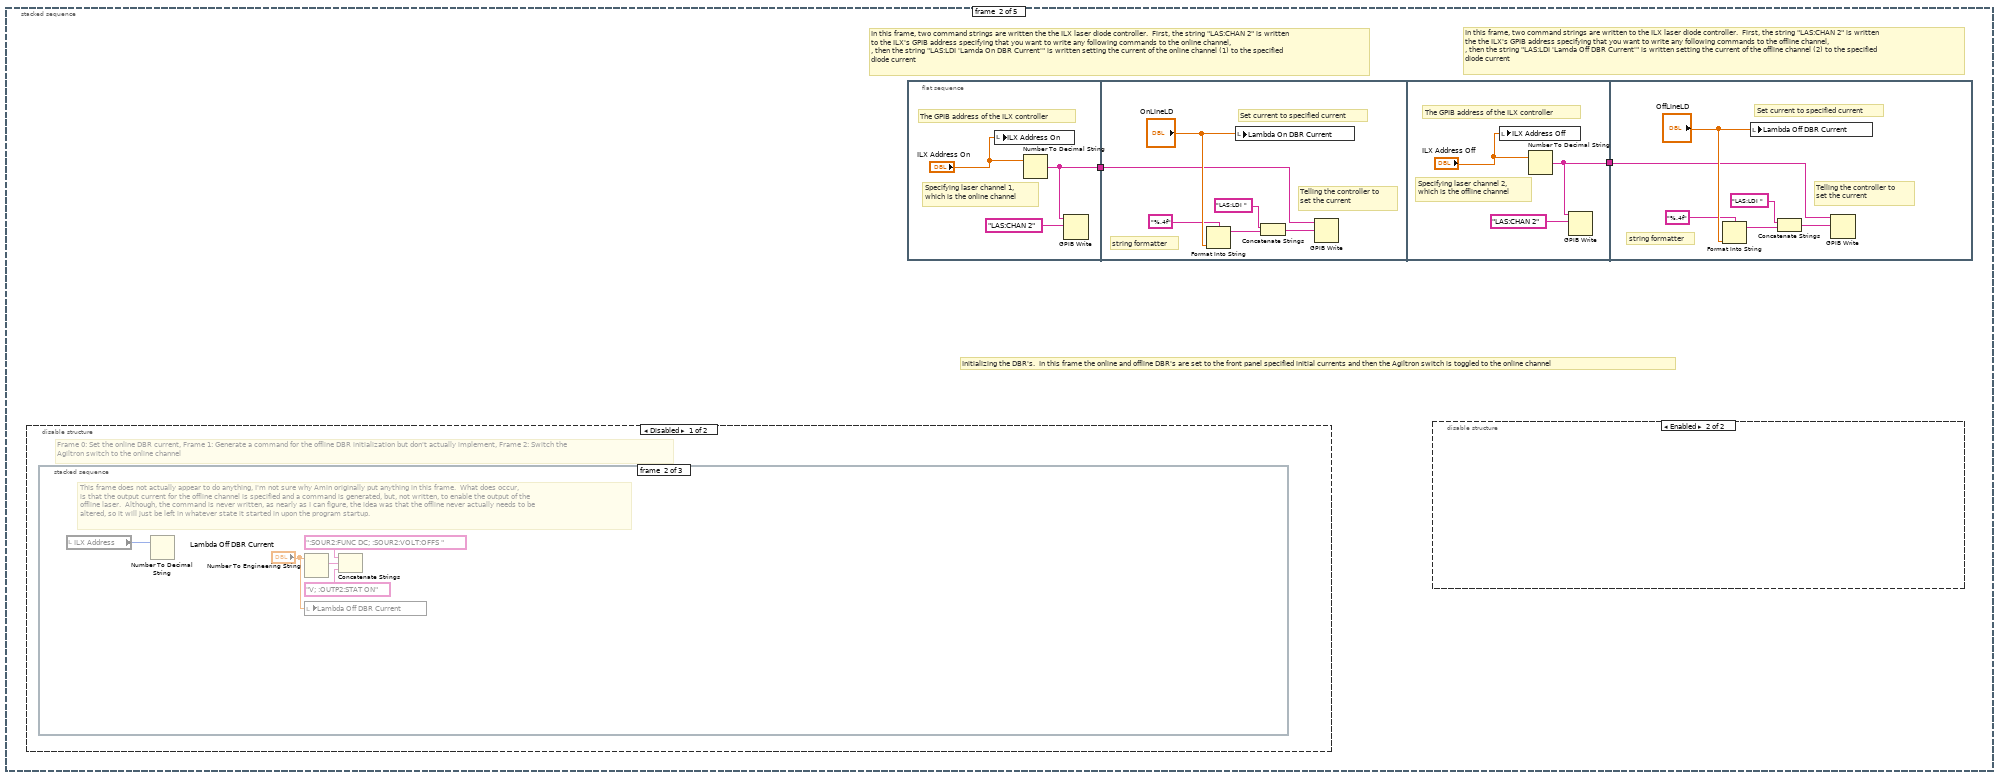
[diagram p5: hidden frame]
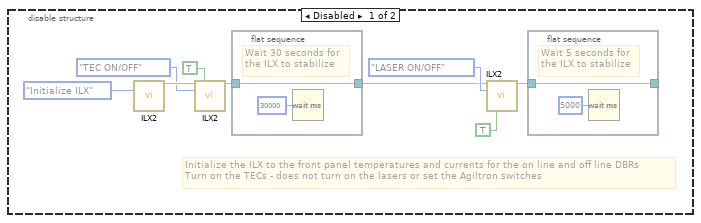
[diagram p6: hidden frame]
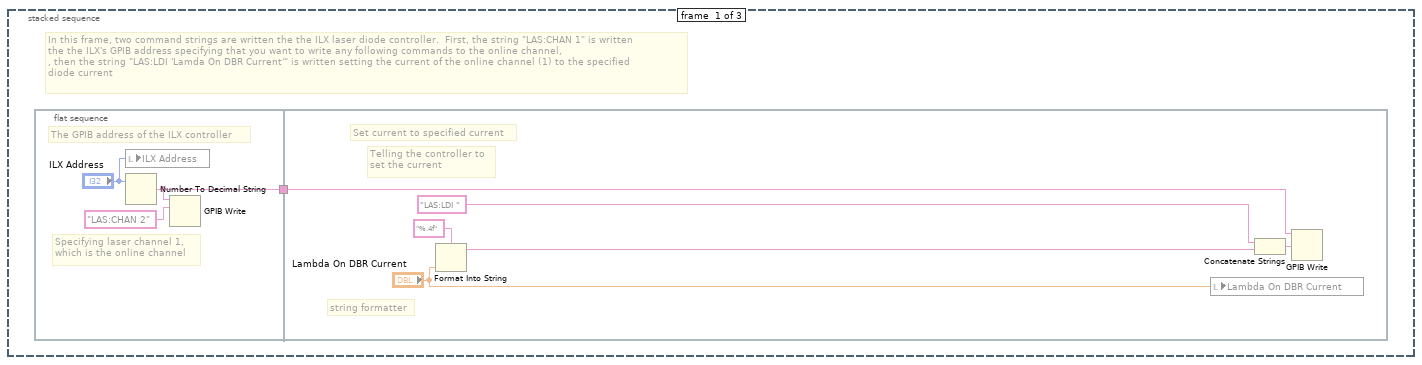
[diagram p7: hidden frame]
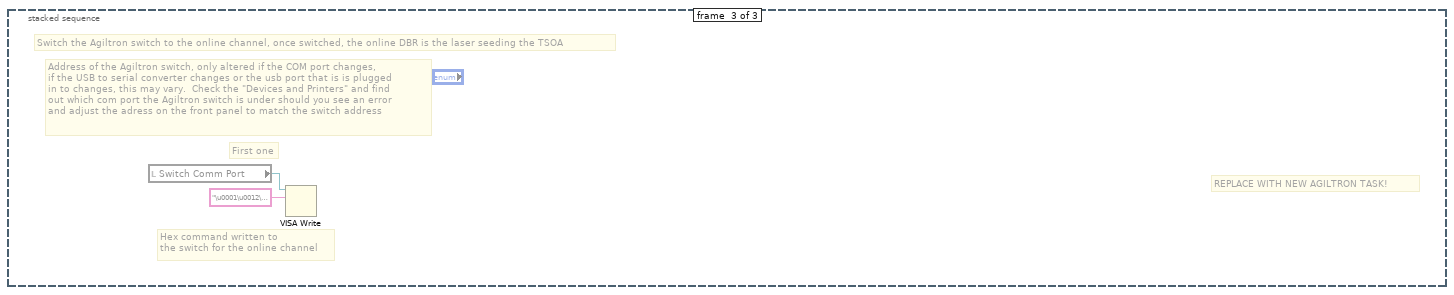
[diagram p8: hidden frame]
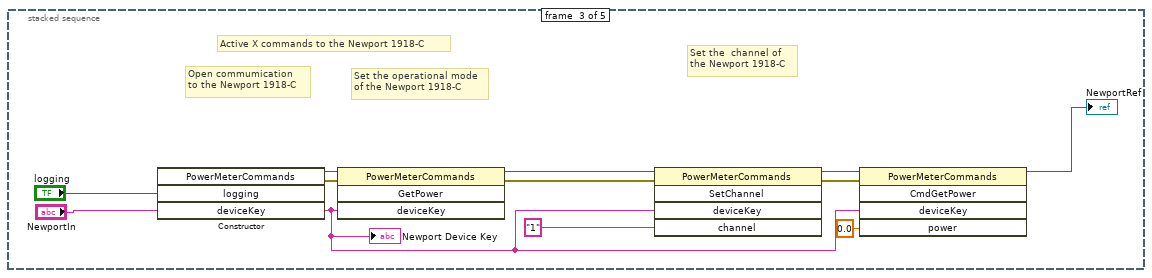
[diagram p10: hidden frame]
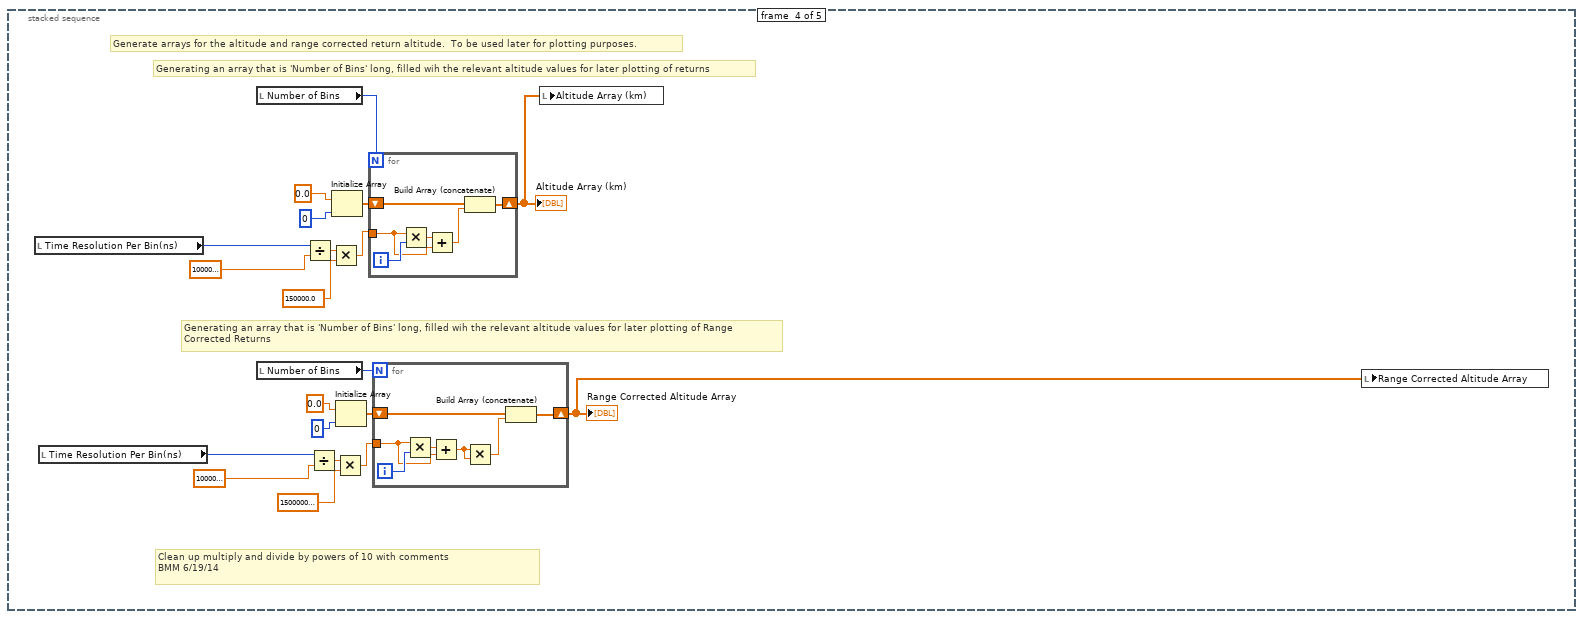
[diagram p11: hidden frame]
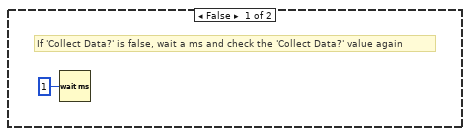
[diagram p12: hidden frame]
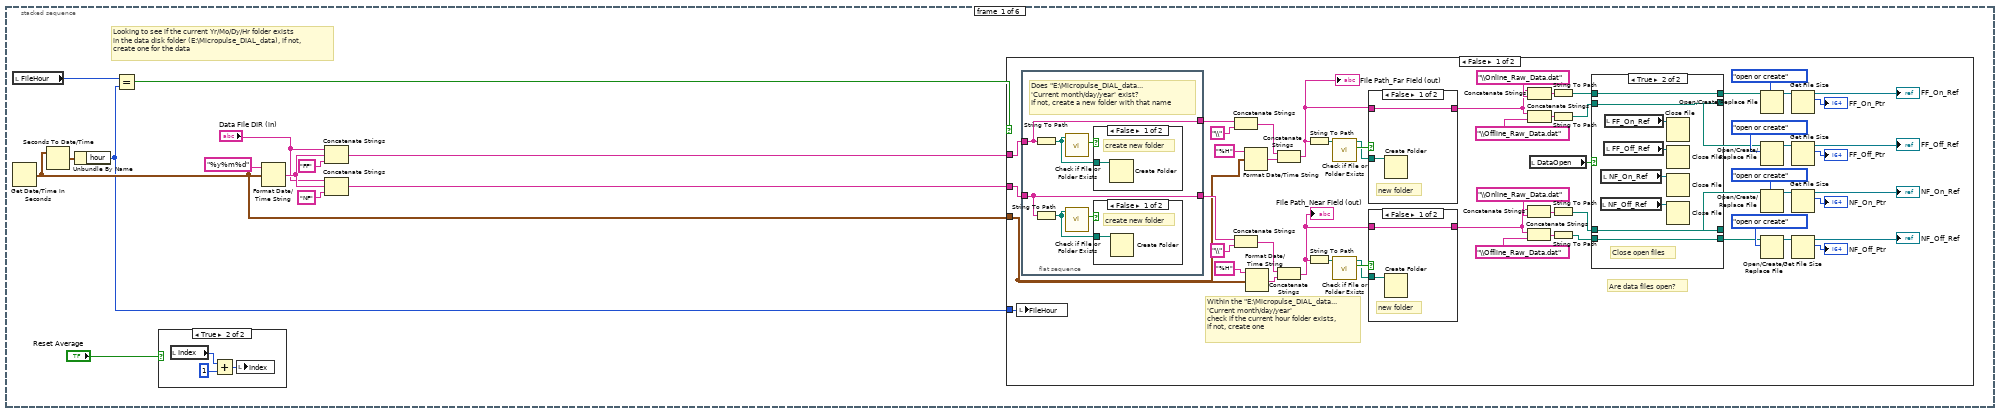
[diagram p13: hidden frame]
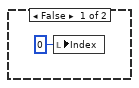
[diagram p20: hidden frame]
diagram:
  # "Frame 0: Initialize the scaler card (and start the MCSC)\nFrame 1: Initialize the DBR's\nFrame 2: Generate address string for talking the to Newport Power meter\nFrame 3: Generate altitude axes for regular and range corrected returns\nFrame 4: Collect data"
  n1 = stacked-sequence {
    tunnel: [_ _ _ _ w125] -> w3
    frame #0 {
      # "Open Bristol WM"
      n2 = disable-structure shown="Enabled" {
        frame Enabled {
          # "Initialization of the AMCS card, this where all of the scaler card parameters\nsuch as number of channels and accumulates is written to the card"
          n3 = stacked-sequence {
            frame #0 {
              # "Sets The Registers Of The Card"
              # "Number Of Channels Used"
              n4 = To Unsigned Long Integer(number="Sync Pulse Polarity") -> (unsigned 32bit integer=w9:u32)
              n5 = To Unsigned Long Integer(number="Pulse A Polarity") -> (unsigned 32bit integer=w13:u32)
              n6 = To Unsigned Long Integer(number="Pulse B Polarity") -> (unsigned 32bit integer=w11:u32)
              n7 = expression code="x*4"(w9) -> (w18:u32)
              n8 = expression code="x*2"(w13) -> (w17:u32)
              n9 = expression code="(x-1)*256"(u32 4 ("Number of Channels Used")) -> (w16:u32)
              n10 = expression code="x/10"("Time Resolution Per Bin(ns)") -> (w20:u32)
              n11 = expression code="x/80"("Pulse A Delay(ns)") -> (w27:u32)
              n12 = expression code="x/80"("Pulse B Delay(ns)") -> (w29:u32)
              n13 = expression code="x/10"("Accumulation Delay(ns)") -> (w28:u32)
              n14 = Compound Arithmetic op=ADD(w18, w17, w11, w16) -> (w15:u32)
              n15 = Build Array(w15, "Number of Bins", "Number of Accumulates", w20, w27, w29, w28) -> ()  [unwired: 1 out]
              n16 = local write "ns scale"("Time Resolution Per Bin(ns)") -> ()
              n17 = local write "y offset"("Accumulation Delay(ns)") -> ()
              n18 = local write "bins"("Number of Bins") -> ()
            }
          }
        }
        frame Disabled {
        }
      }
      n19 = local read "Number of Bins"() -> (w7:u32)
      n20 = Decrement(x=w7) -> (x-1=w6:u32)
      n21 = Subtract(x=w6, y="background length") -> (x-y=→"background start":u32)
      "Index" <- 0 ("Index")
    }
    frame #1 {
      # "In this frame, two command strings are written to the ILX laser diode controller.  First, the string \"LAS:CHAN 2\" is written\nthe the ILX's GPIB address specifying that you want to write any following commands to the offline channel,\n, then the string \"LAS:LDI 'Lamda Off DBR Current'\" is written setting the current of the offline channel (2) to the specified \ndiode current"
      # "In this frame, two command strings are written the the ILX laser diode controller.  First, the string \"LAS:CHAN 2\" is written\nto the ILX's GPIB address specifying that you want to write any following commands to the online channel,\n, then the string \"LAS:LDI 'Lamda On DBR Current'\" is written setting the current of the online channel (1) to the specified \ndiode current"
      # "Initializing the DBR's.  In this frame the online and offline DBR's are set to the front panel specified initial currents and then the Agiltron switch is toggled to the online channel"
      n22 = disable-structure shown="Disabled" {
        frame Disabled {
          # "Frame 0: Set the online DBR current, Frame 1: Generate a command for the offline DBR initialization but don't actually implement, Frame 2: Switch the \nAgiltron switch to the online channel"
          n23 = stacked-sequence {
            frame #0 {
              # "In this frame, two command strings are written the the ILX laser diode controller.  First, the string \"LAS:CHAN 1\" is written\nthe the ILX's GPIB address specifying that you want to write any following commands to the online channel,\n, then the string \"LAS:LDI 'Lamda On DBR Current'\" is written setting the current of the online channel (1) to the specified \ndiode current"
              n24 = flat-sequence {
                tunnel: [w65] -> w63
                tunnel: w63 -> [w67]
                frame #0 {
                  # "The GPIB address of the ILX controller"
                  # "Specifying laser channel 1,\nwhich is the online channel"
                  n25 = local write "ILX Address"("ILX Address") -> ()
                  n26 = Number To Decimal String(number="ILX Address") -> (decimal integer string=w65:string)  [unwired: 1 in]
                  n27 = GPIB Write(0:w65, 1:"LAS:CHAN 2") -> ()  [unwired: 3 in, 2 out]
                }
                frame #1 {
                  # "Telling the controller to\nset the current"
                  # "string formatter"
                  # "Set current to specified current"
                  n28 = Format Into String(format string="%.4f" ("Format String"), "Lambda On DBR Current") -> (resulting string=w70:string)  [unwired: 2 in, 1 out]
                  n29 = local write "Lambda On DBR Current"("Lambda On DBR Current") -> ()
                  n30 = Concatenate Strings("LAS:LDI ", w70) -> (w71:string)
                  n31 = GPIB Write(0:w67, 1:w71) -> ()  [unwired: 3 in, 2 out]
                }
              }
            }
            frame #1 {
              # "This frame does not actually appear to do anything, I'm not sure why Amin originally put anything in this frame.  What does occur, \nis that the output current for the offline channel is specified and a command is generated, but, not written, to enable the output of the\noffline laser.  Although, the command is never written, as nearly as I can figure, the idea was that the offline never actually needs to be \naltered, so it will just be left in whatever state it started in upon the program startup."
              n32 = local read "ILX Address"() -> (w73:i32)
              n33 = Number To Decimal String(number=w73) -> ()  [unwired: 1 in, 1 out]
              n34 = Number To Engineering String(4:"Lambda Off DBR Current") -> (0:w77:string)  [unwired: 3 in]
              n35 = local write "Lambda Off DBR Current"("Lambda Off DBR Current") -> ()
              n36 = Concatenate Strings(":SOUR2:FUNC DC; :SOUR2:VOLT:OFFS ", w77, "V; :OUTP2:STAT ON") -> ()  [unwired: 1 out]
            }
            frame #2 {
              # "REPLACE WITH NEW AGILTRON TASK!"
              # "First one"
              # "Address of the Agiltron switch, only altered if the COM port changes,\nif the USB to serial converter changes or the usb port that is is plugged\nin to changes, this may vary.  Check the \"Devices and Printers\" and find \nout which com port the Agiltron switch is under should you see an error \nand adjust the adress on the front panel to match the switch address"
              # "Hex command written to \nthe switch for the online channel"
              # "Switch the Agiltron switch to the online channel, once switched, the online DBR is the laser seeding the TSOA"
              n37 = local read "Switch Comm Port"() -> (w78:refnum<visa-resource-name>)
              n38 = VISA Write(VISA resource name=w78, write buffer="\u0001\u0012\u0000\u0002") -> ()  [unwired: 1 in, 3 out]
            }
          }
        }
        frame Enabled {
        }
      }
      n39 = flat-sequence {
        tunnel: [w33] -> w31
        tunnel: w31 -> [w35]
        tunnel: [w41] -> w30
        tunnel: w30 -> [w44]
        frame #0 {
          # "The GPIB address of the ILX controller"
          # "Specifying laser channel 1,\nwhich is the online channel"
          n40 = local write "ILX Address On"("ILX Address On") -> ()
          n41 = Number To Decimal String(number="ILX Address On") -> (decimal integer string=w33:string)  [unwired: 1 in]
          n42 = GPIB Write(0:w33, 1:"LAS:CHAN 2") -> ()  [unwired: 3 in, 2 out]
        }
        frame #1 {
          # "Telling the controller to\nset the current"
          # "string formatter"
          # "Set current to specified current"
          n43 = Format Into String(format string="%.4f" ("Format String"), "OnLineLD") -> (resulting string=w38:string)  [unwired: 2 in, 1 out]
          n44 = local write "Lambda On DBR Current"("OnLineLD") -> ()
          n45 = Concatenate Strings("LAS:LDI ", w38) -> (w39:string)
          n46 = GPIB Write(0:w35, 1:w39) -> ()  [unwired: 3 in, 2 out]
        }
        frame #2 {
          # "The GPIB address of the ILX controller"
          # "Specifying laser channel 2,\nwhich is the offline channel"
          n47 = local write "ILX Address Off"("ILX Address Off") -> ()
          n48 = Number To Decimal String(number="ILX Address Off") -> (decimal integer string=w41:string)  [unwired: 1 in]
          n49 = GPIB Write(0:w41, 1:"LAS:CHAN 2") -> ()  [unwired: 3 in, 2 out]
        }
        frame #3 {
          # "Telling the controller to\nset the current"
          # "string formatter"
          # "Set current to specified current"
          n50 = Format Into String(format string="%.4f" ("Format String"), "OffLineLD") -> (resulting string=w47:string)  [unwired: 2 in, 1 out]
          n51 = local write "Lambda Off DBR Current"("OffLineLD") -> ()
          n52 = Concatenate Strings("LAS:LDI ", w47) -> (w48:string)
          n53 = GPIB Write(0:w44, 1:w48) -> ()  [unwired: 3 in, 2 out]
        }
      }
      n54 = disable-structure shown="Enabled" {
        frame Disabled {
          # "Initialize the ILX to the front panel temperatures and currents for the on line and off line DBRs\nTurn on the TECs - does not turn on the lasers or set the Agiltron switches"
          n55 = call "ILX2.vi"("ILX Command"=T6."Initialize ILX") -> ("Device Out"=w57:refnum<visa-resource-name>)  [unwired: 10 in, 4 out]
          n56 = call "ILX2.vi"("Device In"=w57, "TEC Control"=TRUE, "ILX Command"=T6."TEC ON/OFF") -> ("Device Out"=w54:refnum<visa-resource-name>)  [unwired: 8 in, 4 out]
          n57 = flat-sequence {
            tunnel: w54 -> [w61]
            tunnel: [w61] -> w51
            frame #0 {
              # "Wait 30 seconds for\nthe ILX to stabilize"
              n58 = Wait (ms)(milliseconds to wait=u32 30000) -> ()  [unwired: 1 out]
            }
          }
          n59 = call "ILX2.vi"("Device In"=w51, "ILX Command"=T6."LASER ON/OFF", "Laser Control"=TRUE ("TEC Control")) -> ("Device Out"=w50:refnum<visa-resource-name>)  [unwired: 8 in, 4 out]
          n60 = flat-sequence {
            tunnel: w50 -> [w59]
            tunnel: [w59] -> _
            frame #0 {
              # "Wait 5 seconds for\nthe ILX to stabilize"
              n61 = Wait (ms)(milliseconds to wait=u32 5000) -> ()  [unwired: 1 out]
            }
          }
        }
        frame Enabled {
        }
      }
    }
    frame #2 {
      # "Active X commands to the Newport 1918-C"
      # "Set the  channel of\nthe Newport 1918-C"
      # "Set the operational mode\nof the Newport 1918-C"
      # "Open commumication\nto the Newport 1918-C"
      n62 = constructor class="PowerMeterCommands"("logging"="logging", "deviceKey"="NewportIn") -> (reference out=w91:refnum<k24>, error out=w88:errorcluster, "deviceKey"=w83:string)  [unwired: 3 in, 2 out]
      "Newport Device Key" <- w83
      n63 = invoke class="PowerMeterCommands" method="GetPower"(reference=w91, error in=w88, "deviceKey"=w83) -> (reference out=w90:refnum<k24>, error out=w87:errorcluster)  [unwired: 1 in, 2 out]
      n64 = invoke class="PowerMeterCommands" method="SetChannel"(reference=w90, error in=w87, "deviceKey"=w83, "channel"="1") -> (reference out=w84:refnum<k24>, error out=w86:errorcluster)  [unwired: 1 in, 3 out]
      n65 = invoke class="PowerMeterCommands" method="CmdGetPower"(reference=w84, error in=w86, "deviceKey"=w83, "power"=sgl 0.0) -> (reference out=→"NewportRef":refnum<k24>)  [unwired: 1 in, 4 out]
    }
    frame #3 {
      # "Clean up multiply and divide by powers of 10 with comments\nBMM 6/19/14"
      # "Generating an array that is 'Number of Bins' long, filled wih the relevant altitude values for later plotting of Range \nCorrected Returns"
      # "Generating an array that is 'Number of Bins' long, filled wih the relevant altitude values for later plotting of returns"
      # "Generate arrays for the altitude and range corrected return altitude.  To be used later for plotting purposes."
      n66 = local read "Time Resolution Per Bin(ns)"() -> (w104:u32)
      n67 = local read "Time Resolution Per Bin(ns)"() -> (w94:u32)
      n68 = local read "Number of Bins"() -> (w107:u32)
      n69 = local read "Number of Bins"() -> (w97:u32)
      n70 = Divide(x=w104, y=1000000000.0) -> (x/y=w102:dbl)
      n71 = Divide(x=w94, y=1000000000.0) -> (x/y=w92:dbl)
      n72 = Multiply(x=w102, y=150000.0) -> (x*y=w105:dbl)
      n73 = Initialize Array(0.0, 0) -> (w110:dbl[])
      n74 = Multiply(x=w92, y=150000000.0) -> (x*y=w95:dbl)
      n75 = Initialize Array(0.0, 0) -> (w100:dbl[])
      n76 = for {
        N: w107 -> [_]
        shift-right: [w123] -> w108
        shift-left: w110 -> [w124]
        tunnel: w105 -> [w120]
        i -> [w122]
        n77 = Multiply(x=w120, y=w122) -> (x*y=w121:dbl)
        n78 = Add(x=w121, y=w120) -> (x+y=w119:dbl)
        n79 = Build Array (concatenate)(w124, w119) -> (w123:dbl[])
      }
      "Altitude Array (km)" <- w108
      n80 = for {
        N: w97 -> [_]
        shift-right: [w117] -> w98
        shift-left: w100 -> [w118]
        tunnel: w95 -> [w113]
        i -> [w116]
        n81 = Multiply(x=w113, y=w116) -> (x*y=w114:dbl)
        n82 = Add(x=w114, y=w113) -> (x+y=w112:dbl)
        n83 = Multiply(x=w112, y=w112) -> (x*y=w115:dbl)
        n84 = Build Array (concatenate)(w118, w115) -> (w117:dbl[])
      }
      "Range Corrected Altitude Array" <- w98
      n85 = local write "Altitude Array (km)"(w108) -> ()
      n86 = local write "Range Corrected Altitude Array"(w98) -> ()
    }
    frame #4 {
      # "Frame 4: Collect data from the scaler card and process and file it"
      n87 = while {
        tunnel: ["stop"] -> w125
        i -> [w126]
        stop <- "stop" stop-if-true
        # "While loop continues data collection cycle"
        n88 = case shown="True" "Collect Data?" {
          frame False {
            # "If 'Collect Data?' is false, wait a ms and check the 'Collect Data?' value again"
            n89 = Wait (ms)(milliseconds to wait=u32 1) -> ()  [unwired: 1 out]
          }
          frame True {
            # "Frame 3: Read the offline wavelength and lock if necessary (code not finished), read output power, read offline data, perform calculations and plot/save offline and NRB data, switch to online\nFrame 4: Calculate the absorption cross section (if wavelength, T, or P changed)\nFrame 5: Calculate Water Vapor Number density and plot"
            # "Frame 0: Create folders and file paths for logging the data, initialize averaging index\nFrame 1: Import current pressure and temperature data from COE weather station\nFrame 2: Read the online wavelength and lock if necessary, read online data and output power\n, plot and save online data, switch to offline DBR"
            # "If 'Collect Data?' is true, collect, process, and log data"
            n90 = stacked-sequence {
              frame #0 {
                # "Looking to see if the current Yr/Mo/Dy/Hr folder exists\nin the data disk folder (E:\\Micropulse_DIAL_data), if not,\ncreate one for the data"
                n91 = local read "FileHour"() -> (w139:i32)
                n92 = Get Date/Time In Seconds() -> (seconds since 1Jan1904=w131:timestamp)
                n93 = Seconds To Date/Time(time stamp (now)=w131) -> (date time rec=w141:T8)  [unwired: 1 in]
                n94 = Unbundle By Name(w141) -> ("hour"=w130:i32)
                n95 = Equal?(x=w139, y=w130) -> (x = y?=w140:bool)
                n96 = case shown="True" "Reset Average" {
                  frame False {
                    n97 = local write "Index"(0 ("Index")) -> ()
                  }
                  frame True {
                    n98 = local read "Index"() -> (w229:i32)
                    n99 = Add(x=w229, y=1) -> (x+y=w228:i32)
                    n100 = local write "Index"(w228) -> ()
                  }
                }
                n101 = Format Date/Time String(time format string (%c)="%y%m%d", seconds (now)=w131) -> (date/time string=w135:string)  [unwired: 1 in]
                n102 = Concatenate Strings("Data File DIR (in)", w135, "FF" ("string")) -> (w137:string)
                n103 = Concatenate Strings("Data File DIR (in)", w135, "NF" ("string")) -> (w132:string)
                n104 = case shown="False" w140 {
                  tunnel: w137 -> [w199 _]
                  tunnel: w132 -> [w198 _]
                  tunnel: w131 -> [w185 _]
                  tunnel: w130 -> [w161 _]
                  frame False {
                    # "Are data files open?"
                    # "Within the \"E:\\Micropulse_DIAL_data...\n'Current month/day/year' \ncheck if the current hour folder exists,\nif not, create one"
                    n105 = local write "FileHour"(w161) -> ()
                    n106 = flat-sequence {
                      tunnel: [w219] -> w186
                      tunnel: w199 -> [w218]
                      tunnel: w198 -> [w219]
                      tunnel: [w218] -> w187
                      frame #0 {
                        # "Does \"E:\\Micropulse_DIAL_data...\n'Current month/day/year' exist?\nIf not, create a new folder with that name"
                        n107 = String To Path(string=w218) -> (path=w223:path)
                        n108 = String To Path(string=w219) -> (path=w221:path)
                        n109 = call <vilib>:"Check if File or Folder Exists.vi"("path"=w223) -> ("file or folder exists?"=w222:bool)  [unwired: 8 in, 2 out]
                        n110 = call <vilib>:"Check if File or Folder Exists.vi"("path"=w221) -> ("file or folder exists?"=w220:bool)  [unwired: 8 in, 2 out]
                        n111 = case shown="False" w222 {
                          tunnel: w223 -> [w225 _]
                          frame False {
                            # "create new folder"
                            n112 = Create Folder(path (use dialog)=w225) -> ()  [unwired: 2 in, 3 out]
                          }
                          frame True {
                            # "Folder exists\ndo nothing"
                          }
                        }
                        n113 = case shown="False" w220 {
                          tunnel: w221 -> [w224 _]
                          frame False {
                            # "create new folder"
                            n114 = Create Folder(path (use dialog)=w224) -> ()  [unwired: 2 in, 3 out]
                          }
                          frame True {
                            # "Folder exists\ndo nothing"
                          }
                        }
                      }
                    }
                    n115 = Concatenate Strings(w187, "\\" ("string")) -> (w194:string)
                    n116 = Concatenate Strings(w186, "\\" ("string")) -> (w189:string)
                    n117 = Format Date/Time String(time format string (%c)="%H", seconds (now)=w185) -> (date/time string=w197:string)  [unwired: 1 in]
                    n118 = Format Date/Time String(time format string (%c)="%H", seconds (now)=w185) -> (date/time string=w192:string)  [unwired: 1 in]
                    n119 = Concatenate Strings(w194, w197) -> (w157:string)
                    "File Path_Far Field (out)" <- w157
                    n120 = Concatenate Strings(w189, w192) -> (w158:string)
                    "File Path_Near Field (out)" <- w158
                    n121 = String To Path(string=w157) -> (path=w195:path)
                    n122 = String To Path(string=w158) -> (path=w190:path)
                    n123 = call <vilib>:"Check if File or Folder Exists.vi"("path"=w195) -> ("file or folder exists?"=w184:bool, "dup path"=w182:path)  [unwired: 8 in, 1 out]
                    n124 = call <vilib>:"Check if File or Folder Exists.vi"("path"=w190) -> ("file or folder exists?"=w183:bool, "dup path"=w181:path)  [unwired: 8 in, 1 out]
                    n125 = case shown="False" w184 {
                      tunnel: w182 -> [w216 _]
                      tunnel: w157 -> [w215 w217]
                      tunnel: [w215 w217] -> w155
                      frame False {
                        # "new folder"
                        n126 = Create Folder(path (use dialog)=w216) -> ()  [unwired: 2 in, 3 out]
                      }
                      frame True {
                        # "Folder exists\ndo nothing"
                      }
                    }
                    n127 = case shown="False" w183 {
                      tunnel: w181 -> [w213 _]
                      tunnel: w158 -> [w212 w214]
                      tunnel: [w212 w214] -> w156
                      frame False {
                        # "new folder"
                        n128 = Create Folder(path (use dialog)=w213) -> ()  [unwired: 2 in, 3 out]
                      }
                      frame True {
                        # "Folder exists\ndo nothing"
                      }
                    }
                    n129 = Concatenate Strings(w156, "\\Online_Raw_Data.dat" ("string")) -> (w175:string)
                    n130 = Concatenate Strings(w156, "\\Offline_Raw_Data.dat" ("string")) -> (w174:string)
                    n131 = Concatenate Strings(w155, "\\Online_Raw_Data.dat" ("string")) -> (w180:string)
                    n132 = Concatenate Strings(w155, "\\Offline_Raw_Data.dat" ("string")) -> (w179:string)
                    n133 = local read "DataOpen"() -> (w172:bool)
                    n134 = String To Path(string=w180) -> (path=w171:path)
                    n135 = String To Path(string=w179) -> (path=w170:path)
                    n136 = String To Path(string=w175) -> (path=w169:path)
                    n137 = String To Path(string=w174) -> (path=w168:path)
                    n138 = case shown="True" w172 {
                      tunnel: w171 -> [w203 w207]
                      tunnel: [w203 w207] -> w165
                      tunnel: w170 -> [w202 w206]
                      tunnel: [w202 w206] -> w164
                      tunnel: w169 -> [w201 w205]
                      tunnel: [w201 w205] -> w163
                      tunnel: [w200 w204] -> w162
                      tunnel: w168 -> [w200 w204]
                      frame False {
                        # "No files open\ndo nothing"
                      }
                      frame True {
                        # "Close open files"
                        n139 = local read "NF_Off_Ref"() -> (w209:refnum<file>)
                        n140 = local read "NF_On_Ref"() -> (w208:refnum<file>)
                        n141 = local read "FF_Off_Ref"() -> (w211:refnum<file>)
                        n142 = local read "FF_On_Ref"() -> (w210:refnum<file>)
                        n143 = Close File(refnum=w210) -> ()  [unwired: 1 in, 2 out]
                        n144 = Close File(refnum=w211) -> ()  [unwired: 1 in, 2 out]
                        n145 = Close File(refnum=w208) -> ()  [unwired: 1 in, 2 out]
                        n146 = Close File(refnum=w209) -> ()  [unwired: 1 in, 2 out]
                      }
                    }
                    n147 = Open/Create/Replace File(file path (use dialog)=w165, operation (0:open)=T7."open or create") -> (refnum out=w151:refnum<file>)  [unwired: 4 in, 2 out]
                    n148 = Open/Create/Replace File(file path (use dialog)=w164, operation (0:open)=T7."open or create") -> (refnum out=w152:refnum<file>)  [unwired: 4 in, 2 out]
                    n149 = Open/Create/Replace File(file path (use dialog)=w163, operation (0:open)=T7."open or create") -> (refnum out=w153:refnum<file>)  [unwired: 4 in, 2 out]
                    n150 = Open/Create/Replace File(file path (use dialog)=w162, operation (0:open)=T7."open or create") -> (refnum out=w154:refnum<file>)  [unwired: 4 in, 2 out]
                    n151 = Get File Size(file=w151) -> (refnum out=→"FF_On_Ref":refnum<file>, size (in bytes)=→"FF_On_Ptr":i64)  [unwired: 1 in, 1 out]
                    n152 = Get File Size(file=w152) -> (refnum out=→"FF_Off_Ref":refnum<file>, size (in bytes)=→"FF_Off_Ptr":i64)  [unwired: 1 in, 1 out]
                    n153 = Get File Size(file=w153) -> (refnum out=→"NF_On_Ref":refnum<file>, size (in bytes)=→"NF_On_Ptr":i64)  [unwired: 1 in, 1 out]
                    n154 = Get File Size(file=w154) -> (refnum out=→"NF_Off_Ref":refnum<file>, size (in bytes)=→"NF_Off_Ptr":i64)  [unwired: 1 in, 1 out]
                  }
                  frame True {
                    # "Don't need to do anything!"
                  }
                }
              }
              frame #1 {
                # "Writing and plotting retrieved\nweather parameters"
                # "Matlab script goes online and retrieves most recent press, temp, and relative humidity data \nfrom the weather station on the roof of Cobleigh"
                # "Importing the current weather conditions from the COE weather station"
                n155 = disable-structure shown="Disabled" {
                  frame Disabled {
                    n156 = script code="%try\n%s=urlread('http://www.coe.montana.edu/ee/weather/mostCurrentCSV.php');\n%amin=textscan(s,'%s %s %s %s %s %s %s %s %s %s %s %s %s');\n%data=amin{1}{2};\n%[test remain]=strtok(data,',');\n%remain=str2num(remain);\n%press=remain(3)./1000;\n%temp=remain(5);\n%RH=remain(7);\n%catch\npress=.850;\ntemp=20;\nRH=40;\n%end"() -> ()  [unwired: 1 in, 4 out]
                  }
                  frame Enabled {
                  }
                }
                "Temperature (C)" <- "Temperature (C)"
                "Pressure (mb)" <- "Pressure (mbar or hPa)"
                "Relative Humdity (%)" <- 40.0 ("Real")
              }
              frame #2 {
                # "Frame 3: Read, process, and plot online data\nFrame 4:\nFrame 5: Write the data to the folders from Frame 0 of outter sequence"
                # "Frame 0: Read the online wavelength and adjust to locking tolerance if out of range, Switch to offline DBR\nFrame 1: Read the output power from the Newport meter, calculate and plot the output pulse energy\nFrame 2: Wait 'Scalar Wait Time' for buffer to clear other wavelength data"
                # "Online"
                n157 = stacked-sequence {
                  frame #0 {
                    n158 = local read "L_Count"() -> (w235:i32)
                    n159 = Add(x=w235, y=60) -> (x+y=w233:i32)
                    n160 = Quotient & Remainder(x=w233, y=1.0) -> (x-y*floor(x/y)=w237:dbl)  [unwired: 1 out]
                    n161 = Equal To 0?(x=w237) -> (x = 0?=w236:bool)
                    n162 = case shown="True" w236 {
                      frame False {
                      }
                      frame True {
                        # "Read the online wavelength and continue adjusting the online DBR if outside the wavelength tolerance\nuntil it is within tolerance"
                        n163 = flat-sequence {
                          frame #0 {
                            # "Set the TSOA switch to\namplify the ABSORBING\nwavelength"
                            n164 = Build Array(FALSE ("Boolean")) -> (w239:bool[])
                            n165 = call-poly <vilib>:"DAQmx Write.vi"("task/channels in"=refnum<k21> "BristolWM", "data"=w239) -> ()  [unwired: 11 in, 3 out]
                          }
                          frame #1 {
                            n166 = while {
                              stop <- w242 stop-if-true
                              # "If WL difference is within tolerance, stop looping, and illuminate 'Wavelength Lock Online' indicator"
                              # "Frame 2: Decrement DBR current if above tolerance\nFrame 3: Increment DBR current if below tolerance"
                              # "Frame 0: Read the current wavelength from the wavemeter\nFrame 1: Calculate the difference between desired and actual wavelength"
                              # "Continue reading and adjusting online DBR current until within locking tolerance"
                              n167 = local read "AB_DIF"() -> (w245:dbl)
                              n168 = local read "ILX Address On"() -> (w243:dbl)
                              n169 = stacked-sequence {
                                tunnel: w243 -> [_ _ w261 w278]
                                frame #0 {
                                # "Reading the wavelength from the wavemeter"
                                n170 = flat-sequence {
                                tunnel: [w251] -> w250
                                tunnel: w250 -> [w254]
                                tunnel: [w253] -> w249
                                tunnel: w249 -> [w257]
                                frame #0 {
                                n171 = local read "Bristol In"() -> (w252:i32)
                                n172 = dll-call lib="C:/Users/H2ODial/Desktop/Shared Telescope WV DIAL Code/Libraries and VIs/CLDevIface.dll" fn="CLOpenUSBSerialDevice"("commPort"=w252) -> ("return type"=w251:i32)  [unwired: 4 in, 2 out]
                                }
                                frame #1 {
                                n173 = dll-call lib="C:/Users/H2ODial/Desktop/Shared Telescope WV DIAL Code/Libraries and VIs/CLDevIface.dll" fn="CLGetLambdaReading"("devHandle"=w254) -> ("return type"=→"Lambda On Read (nm)":dbl, "devHandle"=w253:i32)  [unwired: 3 in, 2 out]
                                }
                                frame #2 {
                                n174 = dll-call lib="C:/Users/H2ODial/Desktop/Shared Telescope WV DIAL Code/Libraries and VIs/CLDevIface.dll" fn="CLCloseDevice"("commPort"=w257) -> ("return type"=w256:i32)  [unwired: 4 in, 2 out]
                                n175 = local write "Bristol Out"(w256) -> ()
                                }
                                }
                                }
                                frame #1 {
                                # "Calculating the difference between the actual and desired online wavelength"
                                n176 = local read "Lambda On Read (nm)"() -> (w260:dbl)
                                n177 = Subtract(x=w260, y="Lambda On Set (nm)") -> (x-y=→"AB_DIF":dbl)
                                }
                                frame #2 {
                                # "If the wavelength difference is greater that 0.0002 nm, decrement the \nDBR current by 0.01 mA"
                                n178 = local read "AB_DIF"() -> (w264:dbl)
                                n179 = Greater Or Equal?(x=w264, y=0.0001) -> (x >= y?=w262:bool)
                                n180 = case shown="True" w262 {
                                tunnel: w261 -> [_ w265]
                                frame False {
                                # "Wavelength difference is not greater than 0.0002 nm, do nothing"
                                }
                                frame True {
                                n181 = stacked-sequence {
                                tunnel: w265 -> [w266 w269]
                                frame #0 {
                                # "Specifying laser channel 1,\nwhich is the online channel"
                                n182 = Number To Decimal String(number=w266) -> (decimal integer string=w267:string)  [unwired: 1 in]
                                n183 = GPIB Write(0:w267, 1:"LAS:CHAN 2") -> ()  [unwired: 3 in, 2 out]
                                }
                                frame #1 {
                                # "issuing the command"
                                # "Generating a command string\nto decrement the current"
                                # "WL difference is greater than 0.0002 nm,\ndecrement the DBR current by 0.01 mA"
                                n184 = local read "Lambda On DBR Current"() -> (w276:dbl)
                                n185 = Subtract(x=w276, y=0.01) -> (x-y=w270:dbl)
                                n186 = local write "Lambda On DBR Current"(w270) -> ()
                                n187 = Format Into String(format string="%.4f" ("Format String"), w270) -> (resulting string=w273:string)  [unwired: 2 in, 1 out]
                                n188 = Concatenate Strings("LAS:LDI ", w273) -> (w272:string)
                                n189 = Number To Decimal String(number=w269) -> (decimal integer string=w271:string)  [unwired: 1 in]
                                n190 = GPIB Write(0:w271, 1:w272) -> ()  [unwired: 3 in, 2 out]
                                }
                                }
                                }
                                }
                                }
                                frame #3 {
                                # "If WL difference is < 0.0002 nm, increment the DBR current"
                                n191 = local read "AB_DIF"() -> (w281:dbl)
                                n192 = Less Or Equal?(x=w281, y=-0.0001) -> (x <= y?=w279:bool)
                                n193 = case shown="True" w279 {
                                tunnel: w278 -> [_ w282]
                                frame False {
                                # "WL difference is no <= to -0.0002 nm, do nothing"
                                }
                                frame True {
                                n194 = stacked-sequence {
                                tunnel: w282 -> [w284 w286]
                                frame #0 {
                                # "Specifying laser channel 1,\nwhich is the online channel"
                                n195 = Number To Decimal String(number=w284) -> (decimal integer string=w283:string)  [unwired: 1 in]
                                n196 = GPIB Write(0:w283, 1:"LAS:CHAN 2") -> ()  [unwired: 3 in, 2 out]
                                }
                                frame #1 {
                                # "issuing the command"
                                # "Generating a command \nstring to increment the current"
                                # "WL difference is < -0.0002,\nincrement the DBR current by 0.01 mA"
                                n197 = local read "Lambda On DBR Current"() -> (w293:dbl)
                                n198 = Add(x=w293, y=0.01) -> (x+y=w288:dbl)
                                n199 = local write "Lambda On DBR Current"(w288) -> ()
                                n200 = Format Into String(format string="%.4f" ("Format String"), w288) -> (resulting string=w290:string)  [unwired: 2 in, 1 out]
                                n201 = Concatenate Strings("LAS:LDI ", w290) -> (w289:string)
                                n202 = Number To Decimal String(number=w286) -> (decimal integer string=w287:string)  [unwired: 1 in]
                                n203 = GPIB Write(0:w287, 1:w289) -> ()  [unwired: 3 in, 2 out]
                                }
                                }
                                }
                                }
                                }
                              }
                              n204 = Greater?(x=w245, y=-0.00011) -> (0:w247:bool)
                              n205 = Less?(x=w245, y=0.00011) -> (x < y?=w246:bool)
                              n206 = And(x=w247, y=w246) -> (x .and. y?=w242:bool)
                              "Wavelength Lock Online" <- w242
                            }
                          }
                          frame #2 {
                          }
                        }
                      }
                    }
                  }
                  frame #1 {
                    # "Converting to pulse energy, assumes 5 percent pickoff"
                    # "Reading the Newport Power meter"
                    # "Reading the output power of the laser transmitter from the Newport power meter, once read, convert to corresponding pulse energy and plot"
                    n207 = local read "Newport Device Key"() -> (w299:string)
                    n208 = local read "NewportRef"() -> (w295:refnum<k24>)
                    n209 = disable-structure shown="Disabled" {
                      frame Disabled {
                        # "Plotting the online and offling pulse energies"
                        n210 = local read "Online Pulse Energy"() -> (w310:dbl)
                        n211 = local read "Offline Pulse Energy"() -> (w309:dbl)
                        n212 = Bundle("Online Pulse Energy"=w310, "Offline Pulse Energy"=w309) -> (→"Pulse Energy (Micro Joule)":T9)  [unwired: 1 in]
                      }
                      frame Enabled {
                      }
                    }
                    n213 = Number To Decimal String(number="SampleSize") -> (decimal integer string=w297:string)  [unwired: 1 in]
                    n214 = invoke class="PowerMeterCommands" method="PerformDAQ"(reference=w295, "deviceKey"=w299, "interval"="1", "sampleSize"=w297) -> ("PerformDAQ"=w300:dbl[])  [unwired: 2 in, 5 out]
                    n215 = call-poly <vilib>:"Mean.vi"("X"=w300) -> ("mean"=w298:dbl)  [unwired: 1 out]
                    n216 = Multiply(x=w298, y=1000.0) -> (x*y=w306:dbl)
                    n217 = Divide(x=w306, y=0.05) -> (x/y=w304:dbl)
                    n218 = Divide(x=w304, y=7.0) -> (x/y=→"Online Pulse Energy":dbl)
                  }
                  frame #2 {
                    # "Waiting 'Scalar Wait Time'"
                    # "Wait 'Scalar Wait Time' for the next available batch of scalar card data"
                    n219 = Wait (ms)(milliseconds to wait="Scalar Wait Time") -> ()  [unwired: 1 out]
                  }
                  frame #3 {
                    # "convert time per range bin to meters\nand calculate smoothed bins using\nsmoothing range"
                    # "Plotting online cross section and smoothed online data"
                    # "Calculate the bin by bin mean of the data"
                    # "Collect 'Integration Period (Seconds)' number\nof scalar data"
                    # "Reading, processing, and plotting the online data"
                    n220 = local read "Data Reads (number of loops)"() -> (w337:i32)
                    n221 = for {
                      N: w337 -> [_]
                      tunnel: [w358] -> w349 mode=indexing
                      tunnel: [w357] -> w312 mode=indexing
                      # "Scalar Data is retrieved from Global \nVariable that scaler.vi is writing to,"
                      n222 = global read "Scalar_Data.vi" "Scalar Data"() -> (w358:u16[])
                      n223 = global read "Scalar_Data_3.vi" "Scalar Data 3"() -> (w357:u16[])
                    }
                    n224 = Transpose 2D Array(2D array=w349) -> (transposed array=w353:u16[][])
                    n225 = Transpose 2D Array(2D array=w312) -> (transposed array=w335:u16[][])
                    n226 = for {
                      tunnel: w353 -> [w360] mode=indexing
                      tunnel: [w359] -> w354 mode=indexing
                      n227 = call-poly <vilib>:"Mean.vi"("X"=w360) -> ("mean"=w359:dbl)  [unwired: 1 out]
                    }
                    n228 = for {
                      tunnel: w335 -> [w356] mode=indexing
                      tunnel: [w355] -> w336 mode=indexing
                      n229 = call-poly <vilib>:"Mean.vi"("X"=w356) -> ("mean"=w355:dbl)  [unwired: 1 out]
                    }
                    n230 = local read "bins"() -> (w329:u32)
                    n231 = Array Subset(array=w354, index=1 ("dimension size"), length=w329) -> (w341:dbl[])
                    n232 = Array Subset(array=w336, index=1 ("dimension size"), length=w329) -> (w333:dbl[])
                    n233 = local read "background length"() -> (w319:i32)
                    n234 = local read "background start"() -> (w320:u32)
                    n235 = Array Size(array=w341) -> (size(s)=w338:i32)
                    n236 = Array Size(array=w333) -> (size(s)=w330:i32)
                    n237 = Initialize Array(1.0 ("element"), w338) -> (w340:dbl[])
                    n238 = Initialize Array(1.0 ("element"), w330) -> (w332:dbl[])
                    n239 = Multiply(x=w341, y=w340) -> (x*y=w342:dbl[])
                    "On-Line Bin Readings" <- w342
                    n240 = Multiply(x=w333, y=w332) -> (x*y=w323:dbl[])
                    "On-Line Bin Readings 2" <- w323
                    n241 = local read "Total DIAL Integration Time (Minutes)"() -> (w345:i32)
                    n242 = local read "Time Resolution Per Bin(ns)"() -> (w315:u32)
                    n243 = Array Subset(array=w342, index=w320, length=w319) -> (w351:dbl[])
                    n244 = Array Subset(array=w323, index=w320, length=w319) -> (w325:dbl[])
                    n245 = call-poly <vilib>:"Mean.vi"("X"=w351) -> ("mean"=w350:dbl)  [unwired: 1 out]
                    n246 = call-poly <vilib>:"Mean.vi"("X"=w325) -> ("mean"=w326:dbl)  [unwired: 1 out]
                    n247 = Divide(x=w345, y=w337) -> (x/y=w343:dbl)
                    n248 = local read "Index"() -> (w324:i32)
                    n249 = Subtract(x=w342, y=w350) -> (x-y=w347:dbl[])
                    n250 = Subtract(x=w323, y=w326) -> (x-y=w327:dbl[])
                    n251 = To Double Precision Float(number=w315) -> (double precision float=w316:dbl)
                    n252 = Multiply(x=w343, y=60.0) -> (x*y=w321:dbl)
                    n253 = Multiply(x=w316, y=0.15) -> (x*y=w318:dbl)
                    n254 = call "Ring Buffer Online Far.vi"("Index"=w324, "Profiles to Average"=w321, "Input Array"=w347) -> ("AvgArray"=w346:dbl[])  [unwired: 7 in, 1 out]
                    n255 = call "Ring Buffer Online Near.vi"("Index"=w324, "Profiles to Average"=w321, "Input Array"=w327) -> ("AvgArray"=w328:dbl[])  [unwired: 7 in, 1 out]
                    n256 = Divide(x="Smoothing Range", y=w318) -> (x/y=w313:dbl)
                    "Smoothed Bins" <- w313
                    n257 = call "Smooth Arrray.vi"("smooth size"=w313, "Raw Array"=w346) -> ("Smoothed Array"=→"On-Line  Smoothed":dbl[])  [unwired: 9 in]
                    n258 = call "Smooth Arrray.vi"("smooth size"=w313, "Raw Array"=w328) -> ("Smoothed Array"=→"On-Line Smoothed 2":dbl[])  [unwired: 9 in]
                    n259 = disable-structure shown="Disabled" {
                      frame Disabled {
                        n260 = script code="format long;\ncounts=sum(Online);\nif counts >=0.5e6\ntime=time;\nelse\ntime=time\nend"() -> ()  [unwired: 3 in, 2 out]
                      }
                      frame Enabled {
                      }
                    }
                  }
                  frame #4 {
                    # "Toggling the Agiltron switch to the offline DBR seed laser"
                    n261 = disable-structure shown="Disabled" {
                      frame Disabled {
                        n262 = flat-sequence {
                          frame #0 {
                            # "Second one"
                            # "Command the switch to switch to position 2\ncorresponding to the offline DBR"
                            # "Hex string command \ncorrespond to offline"
                            n263 = VISA Write(VISA resource name="Switch Comm Port", write buffer="\u0001\u0012\u0000\u0001") -> ()  [unwired: 1 in, 3 out]
                          }
                        }
                      }
                      frame Enabled {
                      }
                    }
                  }
                  frame #5 {
                    # "Save the recently collected online data if 'Save Data?' is true"
                    n264 = case shown="True" "Save Data?" {
                      frame False {
                        # "'Save Data?' is false, do nothing"
                      }
                      frame True {
                        # "'Save Data?' is true, save onfline data to the Data Disk"
                        # "Write only one copy of data at this time"
                        # "Retrieve Julian Date"
                        n265 = local read "Lambda On DBR Current"() -> (w388:dbl)
                        n266 = local read "Lambda On Read (nm)"() -> (w389:dbl)
                        n267 = local read "On-Line Bin Readings 2"() -> (w383:dbl[])
                        n268 = local read "Relative Humdity (%)"() -> (w384:dbl)
                        n269 = local read "On-Line Bin Readings"() -> (w391:dbl[])
                        n270 = local read "Online Pulse Energy"() -> (w387:dbl)
                        n271 = local read "Temperature (C)"() -> (w386:dbl)
                        n272 = local read "Pressure (mb)"() -> (w385:dbl)
                        n273 = call "Julian_Date_2.vi"() -> ("Julian Date"=w390:dbl)  [unwired: 11 in]
                        n274 = Build Array (concatenate)(w390, w389, w388, w387, w386, w385, w384, w391) -> (w378:dbl[])
                        n275 = Build Array (concatenate)(w390, w389, w388, w387, w386, w385, w384, w383) -> (w368:dbl[])
                        n276 = local write "DataOpen"(TRUE ("DataOpen")) -> ()
                        n277 = local read "NF_On_Ref"() -> (w366:refnum<file>)
                        n278 = local read "FF_On_Ref"() -> (w382:refnum<file>)
                        n279 = local read "NF_On_Ptr"() -> (w367:i64)
                        n280 = local read "FF_On_Ptr"() -> (w381:i64)
                        n281 = Set File Position(offset (in bytes) (0)=w381, refnum=w382) -> (refnum out=w379:refnum<file>, error out=w376:errorcluster)  [unwired: 2 in]
                        n282 = Set File Position(offset (in bytes) (0)=w367, refnum=w366) -> (refnum out=w372:refnum<file>, error out=w370:errorcluster)  [unwired: 2 in]
                        n283 = Write to Binary File(file (use dialog)=w372, data=w368, error in=w370, 5:FALSE ("prepend array or string size? (T)")) -> (refnum out=w371:refnum<file>, error out=w369:errorcluster)  [unwired: 2 in, 1 out]
                        n284 = Write to Binary File(file (use dialog)=w379, data=w378, error in=w376, 5:FALSE ("prepend array or string size? (T)")) -> (refnum out=w377:refnum<file>, error out=w375:errorcluster)  [unwired: 2 in, 1 out]
                        n285 = Get File Position(4:w369, 7:w371) -> (2:w365:i64)  [unwired: 2 out]
                        n286 = Get File Position(4:w375, 7:w377) -> (2:w374:i64)  [unwired: 2 out]
                        n287 = local write "NF_On_Ptr"(w365) -> ()
                        n288 = local write "FF_On_Ptr"(w374) -> ()
                      }
                    }
                  }
                }
              }
              frame #3 {
                # "Frame 3: Read offline data, calculate aerosol data, and plot offline and normalized relative backscatter\nFrame 4:\nFrame 5: Save the offline data and related information"
                # "Frame 0: Read the offline wavelength and lock if necessary, Switch to online DBR\nFrame 1: Read the output power from the Newport power meter\nFrame 2: Wait 'Scalar Wait Time' for buffers to clear of online contiminated data"
                # "offline"
                n289 = stacked-sequence {
                  frame #0 {
                    # "Every 60 data collection cycles, read the offline DBR wavelength, and if outside of wavelength tolerance, adjust DBR current until within tolerance"
                    n290 = local read "L_Count"() -> (w393:i32)
                    n291 = Quotient & Remainder(x=w393, y=60.0) -> (x-y*floor(x/y)=w394:dbl)  [unwired: 1 out]
                    n292 = Equal To 0?(x=w394) -> (x = 0?=w392:bool)
                    n293 = case shown="True" w392 {
                      frame False {
                      }
                      frame True {
                        n294 = flat-sequence {
                          frame #0 {
                            # "Set the TSOA switch to\namplify the non ABSORBING\nwavelength"
                            n295 = Build Array(TRUE ("Boolean")) -> (w396:bool[])
                            n296 = call-poly <vilib>:"DAQmx Write.vi"("task/channels in"=refnum<k21> "BristolWM", "data"=w396) -> ()  [unwired: 11 in, 3 out]
                          }
                          frame #1 {
                            n297 = while {
                              stop <- w399 stop-if-true
                              # "If WL difference is within tolerance, stop looping, and illuminate 'Wavelength Lock Offline' indicator"
                              # "Frame 2: Decrement DBR current if above tolerance\nFrame 3: Increment DBR current if below tolerance"
                              # "Frame 0: Read the current wavelength from the wavemeter\nFrame 1: Calculate the difference between desired and actual wavelength"
                              # "Continue reading and adjusting offline DBR current until within locking tolerance"
                              n298 = local read "NONAB_DIF"() -> (w402:dbl)
                              n299 = local read "ILX Address Off"() -> (w400:dbl)
                              n300 = stacked-sequence {
                                tunnel: w400 -> [_ _ w418 w435]
                                frame #0 {
                                # "Reading the wavelength from the wavemeter"
                                n301 = flat-sequence {
                                tunnel: [w408] -> w407
                                tunnel: w407 -> [w411]
                                tunnel: [w410] -> w406
                                tunnel: w406 -> [w414]
                                frame #0 {
                                n302 = local read "Bristol In"() -> (w409:i32)
                                n303 = dll-call lib="C:/Users/H2ODial/Desktop/Shared Telescope WV DIAL Code/Libraries and VIs/CLDevIface.dll" fn="CLOpenUSBSerialDevice"("commPort"=w409) -> ("return type"=w408:i32)  [unwired: 4 in, 2 out]
                                }
                                frame #1 {
                                n304 = dll-call lib="C:/Users/H2ODial/Desktop/Shared Telescope WV DIAL Code/Libraries and VIs/CLDevIface.dll" fn="CLGetLambdaReading"("devHandle"=w411) -> ("return type"=→"Lambda Off Read (nm)":dbl, "devHandle"=w410:i32)  [unwired: 3 in, 2 out]
                                }
                                frame #2 {
                                n305 = dll-call lib="C:/Users/H2ODial/Desktop/Shared Telescope WV DIAL Code/Libraries and VIs/CLDevIface.dll" fn="CLCloseDevice"("commPort"=w414) -> ("return type"=w413:i32)  [unwired: 4 in, 2 out]
                                n306 = local write "Bristol Out"(w413) -> ()
                                }
                                }
                                }
                                frame #1 {
                                # "Calculating the difference between the actual and desired online wavelength"
                                n307 = local read "Lambda Off Read (nm)"() -> (w417:dbl)
                                n308 = Subtract(x=w417, y="Lambda Off Set (nm)") -> (x-y=→"NONAB_DIF":dbl)
                                }
                                frame #2 {
                                # "If the wavelength difference is greater that 0.0002 nm, decrement the \nDBR current by 0.01 mA"
                                n309 = local read "NONAB_DIF"() -> (w421:dbl)
                                n310 = Greater Or Equal?(x=w421, y=0.0001) -> (x >= y?=w419:bool)
                                n311 = case shown="True" w419 {
                                tunnel: w418 -> [_ w422]
                                frame False {
                                # "Wavelength difference is not greater than 0.0002 nm, do nothing"
                                }
                                frame True {
                                n312 = stacked-sequence {
                                tunnel: w422 -> [w423 w426]
                                frame #0 {
                                # "Specifying laser channel 1,\nwhich is the online channel"
                                n313 = Number To Decimal String(number=w423) -> (decimal integer string=w424:string)  [unwired: 1 in]
                                n314 = GPIB Write(0:w424, 1:"LAS:CHAN 2") -> ()  [unwired: 3 in, 2 out]
                                }
                                frame #1 {
                                # "issuing the command"
                                # "Generating a command string\nto decrement the current"
                                # "WL difference is greater than 0.0002 nm,\ndecrement the DBR current by 0.01 mA"
                                n315 = local read "Lambda Off DBR Current"() -> (w433:dbl)
                                n316 = Subtract(x=w433, y=0.01) -> (x-y=w427:dbl)
                                n317 = local write "Lambda Off DBR Current"(w427) -> ()
                                n318 = Format Into String(format string="%.4f" ("Format String"), w427) -> (resulting string=w430:string)  [unwired: 2 in, 1 out]
                                n319 = Concatenate Strings("LAS:LDI ", w430) -> (w429:string)
                                n320 = Number To Decimal String(number=w426) -> (decimal integer string=w428:string)  [unwired: 1 in]
                                n321 = GPIB Write(0:w428, 1:w429) -> ()  [unwired: 3 in, 2 out]
                                }
                                }
                                }
                                }
                                }
                                frame #3 {
                                # "If WL difference is < 0.0002 nm, increment the DBR current"
                                n322 = local read "NONAB_DIF"() -> (w438:dbl)
                                n323 = Less Or Equal?(x=w438, y=-0.0001) -> (x <= y?=w436:bool)
                                n324 = case shown="True" w436 {
                                tunnel: w435 -> [_ w439]
                                frame False {
                                # "WL difference is no <= to -0.0002 nm, do nothing"
                                }
                                frame True {
                                n325 = stacked-sequence {
                                tunnel: w439 -> [w441 w443]
                                frame #0 {
                                # "Specifying laser channel 1,\nwhich is the online channel"
                                n326 = Number To Decimal String(number=w441) -> (decimal integer string=w440:string)  [unwired: 1 in]
                                n327 = GPIB Write(0:w440, 1:"LAS:CHAN 2") -> ()  [unwired: 3 in, 2 out]
                                }
                                frame #1 {
                                # "issuing the command"
                                # "Generating a command \nstring to increment the current"
                                # "WL difference is < -0.0002,\nincrement the DBR current by 0.01 mA"
                                n328 = local read "Lambda Off DBR Current"() -> (w450:dbl)
                                n329 = Add(x=w450, y=0.01) -> (x+y=w445:dbl)
                                n330 = local write "Lambda Off DBR Current"(w445) -> ()
                                n331 = Format Into String(format string="%.4f" ("Format String"), w445) -> (resulting string=w447:string)  [unwired: 2 in, 1 out]
                                n332 = Concatenate Strings("LAS:LDI ", w447) -> (w446:string)
                                n333 = Number To Decimal String(number=w443) -> (decimal integer string=w444:string)  [unwired: 1 in]
                                n334 = GPIB Write(0:w444, 1:w446) -> ()  [unwired: 3 in, 2 out]
                                }
                                }
                                }
                                }
                                }
                              }
                              n335 = Greater?(x=w402, y=-0.00011) -> (0:w404:bool)
                              n336 = Less?(x=w402, y=0.00011) -> (x < y?=w403:bool)
                              n337 = And(x=w404, y=w403) -> (x .and. y?=w399:bool)
                              "Wavelength Lock Offline" <- w399
                            }
                          }
                          frame #2 {
                            # "Set the TSOA switch to\namplify the ABSORBING\nwavelength"
                            n338 = Build Array(FALSE ("Boolean")) -> (w452:bool[])
                            n339 = call-poly <vilib>:"DAQmx Write.vi"("task/channels in"=refnum<k21> "BristolWM", "data"=w452) -> ()  [unwired: 11 in, 3 out]
                          }
                        }
                      }
                    }
                  }
                  frame #1 {
                    # "Reading the power meter"
                    # "Updating the pulse energy plot"
                    # "Converting to pulse energy"
                    # "Reading the offline output power, converting to pulse energy,  and updating the Pulse energy plot"
                    n340 = local read "SampleSize"() -> (w457:i32)
                    n341 = local read "Newport Device Key"() -> (w458:string)
                    n342 = local read "Online Pulse Energy"() -> (w464:dbl)
                    n343 = local read "Offline Pulse Energy"() -> (w463:dbl)
                    n344 = local read "NewportRef"() -> (w455:refnum<k24>)
                    n345 = Number To Decimal String(number=w457) -> (decimal integer string=w459:string)  [unwired: 1 in]
                    n346 = invoke class="PowerMeterCommands" method="PerformDAQ"(reference=w455, "deviceKey"=w458, "interval"="1", "sampleSize"=w459) -> ("PerformDAQ"=w460:dbl[])  [unwired: 2 in, 5 out]
                    n347 = Bundle("Online Pulse Energy"=w464, "Offline Pulse Energy"=w463) -> (w462:T9)  [unwired: 1 in]
                    n348 = local write "Pulse Energy (Micro Joule)"(w462) -> ()
                    n349 = call-poly <vilib>:"Mean.vi"("X"=w460) -> ("mean"=w456:dbl)  [unwired: 1 out]
                    n350 = Multiply(x=w456, y=1000.0) -> (x*y=w469:dbl)
                    n351 = Divide(x=w469, y=0.05) -> (x/y=w467:dbl)
                    n352 = Divide(x=w467, y=7.0) -> (x/y=→"Offline Pulse Energy":dbl)
                  }
                  frame #2 {
                    # "Wait 'Scalar Wait Time' for buffers to clear of online contiminated offline data"
                    n353 = disable-structure shown="Disabled" {
                      frame Disabled {
                        # "Wait 'Scalar Wait Time'"
                        n354 = local read "Scalar Wait Time"() -> (w471:u32)
                        n355 = Wait (ms)(milliseconds to wait=w471) -> ()  [unwired: 1 out]
                      }
                      frame Enabled {
                      }
                    }
                  }
                  frame #3 {
                    w505 = 1 ("dimension size")
                    w509 = 1
                    # "Plotting the normalized relative \nbackscatter"
                    # "Calculating the normalized relative backscatter"
                    # "Calculating/Plotting smoothed data,\ncross sections etc."
                    # "Pick off data with\nout header"
                    # "Calculate mean bin by bin mean"
                    # "Reading in 'Integration Period (Seconds)' of data"
                    # "Read the offline data from the scalar card, perform smoothing, calculate normalized relative backscatter, and plot"
                    # "File path in MATLAB script is of old dial is:\nF:\\Micropulse DIAL\\Micropulse DIAL Matlab\\\nFinal Overlap Function.mat')];"
                    # "Collects Data From Card,\nSends It To The Chart,\nAnd Saves A Copy As A\nFile If Option Selected On\nFront Panel"
                    n356 = for {
                      N: "Data Reads (number of loops)" -> [_]
                      tunnel: [w541] -> w473 mode=indexing
                      tunnel: [w540] -> w472 mode=indexing
                      # "Read in latest scalar card data from \n'Scalar Data' global variable that \nscaler.vi is writing to, then wait 1 sec\nfor next batch of data"
                      n357 = global read "Scalar_Data_2.vi" "Scalar Data 2"() -> (w541:u16[])
                      n358 = global read "Scalar_Data_4.vi" "Scalar Data 4"() -> (w540:u16[])
                    }
                    n359 = local read "Total DIAL Integration Time (Minutes)"() -> (w530:i32)
                    n360 = Divide(x=w530, y="Data Reads (number of loops)") -> (x/y=w528:dbl)
                    n361 = local read "Total Aerosol Integration Time (Minutes)"() -> (w532:dbl)
                    n362 = local read "background length"() -> (w477:i32)
                    n363 = Multiply(x=w528, y=60.0) -> (x*y=w515:dbl)
                    n364 = local read "background start"() -> (w478:u32)
                    n365 = Transpose 2D Array(2D array=w473) -> (transposed array=w538:u16[][])
                    n366 = Transpose 2D Array(2D array=w472) -> (transposed array=w521:u16[][])
                    n367 = Divide(x=w532, y="Data Reads (number of loops)") -> (x/y=w533:dbl)
                    n368 = for {
                      tunnel: w538 -> [w545] mode=indexing
                      tunnel: [w544] -> w539 mode=indexing
                      tunnel: w521 -> [w543] mode=indexing
                      tunnel: [w542] -> _ mode=indexing
                      tunnel: [w542] -> w518 mode=indexing
                      n369 = call-poly <vilib>:"Mean.vi"("X"=w545) -> ("mean"=w544:dbl)  [unwired: 1 out]
                      n370 = call-poly <vilib>:"Mean.vi"("X"=w543) -> ("mean"=w542:dbl)  [unwired: 1 out]
                    }
                    n371 = local read "bins"() -> (w506:u32)
                    n372 = Multiply(x=w533, y=60.0) -> (x*y=w496:dbl)
                    n373 = Array Subset(array=w518, index=w505, length=w506) -> (w519:dbl[])
                    "Off-Line Bin Readings 2" <- w519
                    n374 = Array Subset(array=w539, index=w505, length=w506) -> (w517:dbl[])
                    "Off-Line  Bin Readings" <- w517
                    n375 = Array Subset(array=w519, index=w478, length=w477) -> (w520:dbl[])
                    n376 = Array Subset(array=w517, index=w478, length=w477) -> (w537:dbl[])
                    n377 = local read "Smoothed Bins"() -> (w474:dbl)
                    n378 = call-poly <vilib>:"Mean.vi"("X"=w520) -> ("mean"=w484:dbl)  [unwired: 1 out]
                    n379 = call-poly <vilib>:"Mean.vi"("X"=w537) -> ("mean"=w485:dbl)  [unwired: 1 out]
                    n380 = local read "Index"() -> (w495:i32)
                    n381 = Subtract(x=w519, y=w484) -> (x-y=w497:dbl[])
                    n382 = Subtract(x=w517, y=w485) -> (x-y=w513:dbl[])
                    n383 = call "Ring Buffer Offline Far.vi"("Index"=w495, "Profiles to Average"=w515, "Input Array"=w513) -> ("AvgArray"=w535:dbl[], "RingBufferOut"=→"RingBuffer offline far":dbl[][])  [unwired: 7 in]
                    n384 = call "Ring Buffer Aerosol Far.vi"("Index"=w495, "Profiles to Average"=w496, "Input Array"=w513) -> ("AvgArray"=w531:dbl[], "RingBufferOut"=→"RingBuffer aerosol far":dbl[][])  [unwired: 7 in]
                    n385 = call "Ring Buffer Offline Near.vi"("Index"=w495, "Profiles to Average"=w515, "Input Array"=w497) -> ("AvgArray"=w516:dbl[], "RingBufferOut"=→"RingBuffer offline near":dbl[][])  [unwired: 7 in]
                    n386 = call "Ring Buffer Aerosol Near.vi"("Index"=w495, "Profiles to Average"=w496, "Input Array"=w497) -> ("AvgArray"=w493:dbl[], "RingBufferOut"=→"RingBuffer aerosol near":dbl[][])  [unwired: 7 in]
                    n387 = Reshape Array(w513, w505, w506) -> (→"raw counts":dbl[][])
                    n388 = Reshape Array(w497, w505, w506) -> (→"raw counts near":dbl[][])
                    n389 = call "Smooth Arrray.vi"("smooth size"=w474, "Raw Array"=w535) -> ("Smoothed Array"=→"Off-Line Smoothed":dbl[])  [unwired: 9 in]
                    n390 = call "Smooth Arrray.vi"("smooth size"=w474, "Raw Array"=w531) -> ("Smoothed Array"=w504:dbl[])  [unwired: 9 in]
                    "Aerosol Smoothed" <- w504
                    n391 = call "Smooth Arrray.vi"("smooth size"=w474, "Raw Array"=w516) -> ("Smoothed Array"=→"Off-Line Smoothed 2":dbl[])  [unwired: 9 in]
                    n392 = call "Smooth Arrray.vi"("smooth size"=w474, "Raw Array"=w493) -> ("Smoothed Array"=w476:dbl[])  [unwired: 9 in]
                    "Aerosol Smoothed 2" <- w476
                    n393 = local read "Number of Accumulates"() -> (w480:u32)
                    n394 = local read "Temperature (C)"() -> (w527:dbl)
                    n395 = local read "Pressure (mb)"() -> (w526:dbl)
                    n396 = script code="%accum_num=10000;     % scaler card setting number of accumulations\nt_bin = 500e-9                 % scaler card setting time per bin\n%t_d = 37.3e-9;                % APD dead time from spec sheet\n\n% conversion from accumulated counts to count rate  (c/s)\nc_convert = 1./t_bin./accum_num;\nCR_far = p_raw_far.*c_convert;\nCR_near = p_raw_near.*c_convert;\nCR_total_far = (p_raw_far+b_far).*c_convert;\nCR_total_near = (p_raw_near+b_near).*c_convert;\nb_CR_far =b_far.*c_convert;\nb_CR_near =b_near.*c_convert;\n\n% create a range array\nsize_p =  size(p_raw_far,2);\nr = (75:75:size_p*75)./1e3; \n    \n%APD correction factor\n D_far = 1./(1-(t_d*CR_total_far));\n D_near = 1./(1-(t_d*CR_total_near));\n\n %Calculating normalize relative backscatter profile\n nrb_far = CR_far.*D_far.*r.^2./E.*1e-6;\n nrb_near = CR_near.*D_near.*r.^2./E.*1e-6;"("E"=6.0 ("Real"), "temp"=w527, "press"=w526, "p_raw_far"=w504, "b_far"=w485, "b_near"=w484, "p_raw_near"=w476, "accum_num"=w480, "t_d"="dead time") -> ("nrb_far"=w499:cdb[], "D_far"=w490:dbl[], "nrb_near"=w498:cdb[], "D_near"=w489:dbl[], "b_CR_far"=w482:dbl, "b_CR_near"=w481:dbl)  [unwired: 1 in, 1 out]
                    n397 = local read "bins"() -> (w508:u32)
                    n398 = local read "Altitude Array (km)"() -> (w501:dbl[])
                    n399 = Bundle(w482, w481) -> (→"?":cluster{dbl, dbl})  [unwired: 1 in]
                    n400 = Build Array(w499, w498) -> (w503:cdb[][])
                    n401 = Build Array(w490, w489) -> (w488:dbl[][])
                    n402 = Reshape Array(w498, w509, w508) -> (→"NRB 2":cdb[][])
                    n403 = Reshape Array(w499, w509, w508) -> (→"NRB":cdb[][])
                    n404 = Build Array(w501, w501) -> (w500:dbl[][])
                    n405 = call "Convert to Dynamic Data7"("2D Array"=w488) -> ("Dynamic Data Type"=w487:dynamicdata)  [unwired: 3 in]
                    n406 = call "Convert to Dynamic Data3"("2D Array"=w503) -> ("Dynamic Data Type"=w502:dynamicdata)  [unwired: 3 in]
                    n407 = call "Convert to Dynamic Data4"("2D Array"=w500) -> ("Dynamic Data Type"=w491:dynamicdata)  [unwired: 3 in]
                    n408 = call "Build XY Graph2"("Y Input"=w491, "X Input"=w502) -> ("XY Graph"=→"NRB plot":cluster{"Y":dbl[], "Y":dbl[]}[])  [unwired: 3 in, 6 out]
                    n409 = call "Build XY Graph4"("Y Input"=w491, "X Input"=w487) -> ("XY Graph"=→"Correction":cluster{"Y":dbl[], "Y":dbl[]}[])  [unwired: 3 in, 6 out]
                  }
                  frame #4 {
                    # "REPLACE WITH NEW AGILTRON TASK!"
                    # "Toggle Agiltron switch to online DBR"
                    n410 = disable-structure shown="Disabled" {
                      frame Disabled {
                        # "ABSORBING"
                        n411 = flat-sequence {
                          frame #0 {
                            # "Third one"
                            # "Command the switch to switch to position 1\ncorresponding to the online DBR"
                            # "Hex string command \ncorrespond to online"
                            n412 = local read "Switch Comm Port"() -> (w549:refnum<visa-resource-name>)
                            n413 = VISA Write(VISA resource name=w549, write buffer="\u0001\u0012\u0000\u0002") -> ()  [unwired: 1 in, 3 out]
                          }
                        }
                        n414 = Build Array(FALSE ("Boolean")) -> (w548:bool[])
                        n415 = call-poly <vilib>:"DAQmx Write.vi"("task/channels in"=refnum<k21> "AgiltronSwitch", "data"=w548) -> ()  [unwired: 11 in, 3 out]
                      }
                      frame Enabled {
                      }
                    }
                  }
                  frame #5 {
                    # "If 'Save Data?' is true, save all relavant offline info"
                    n416 = local read "Save Data?"() -> (w551:bool)
                    n417 = case shown="True" w551 {
                      frame False {
                        # "'Save Data?' is false, do nothing"
                      }
                      frame True {
                        # "Write only one data file at this time"
                        # "Retrive Julian Date"
                        # "'Save Data?' is true, save offline data to the Data Disk"
                        n418 = local read "Lambda Off DBR Current"() -> (w573:dbl)
                        n419 = local read "Off-Line Bin Readings 2"() -> (w570:dbl[])
                        n420 = local read "Lambda Off Read (nm)"() -> (w572:dbl)
                        n421 = local read "Off-Line  Bin Readings"() -> (w578:dbl[])
                        n422 = local read "Relative Humdity (%)"() -> (w577:dbl)
                        n423 = local read "Offline Pulse Energy"() -> (w574:dbl)
                        n424 = local read "Temperature (C)"() -> (w575:dbl)
                        n425 = local read "Pressure (mb)"() -> (w576:dbl)
                        n426 = call "Julian_Date_2.vi"() -> ("Julian Date"=w571:dbl)  [unwired: 11 in]
                        n427 = Build Array (concatenate)(w571, w572, w573, w574, w575, w576, w577, w578) -> (w556:dbl[])
                        n428 = Build Array (concatenate)(w571, w572, w573, w574, w575, w576, w577, w570) -> (w553:dbl[])
                        n429 = local read "FF_Off_Ref"() -> (w558:refnum<file>)
                        n430 = local read "NF_Off_Ref"() -> (w555:refnum<file>)
                        n431 = local read "FF_Off_Ptr"() -> (w557:i64)
                        n432 = local read "NF_Off_Ptr"() -> (w554:i64)
                        n433 = Set File Position(offset (in bytes) (0)=w557, refnum=w558) -> (refnum out=w569:refnum<file>, error out=w567:errorcluster)  [unwired: 2 in]
                        n434 = Set File Position(offset (in bytes) (0)=w554, refnum=w555) -> (refnum out=w565:refnum<file>, error out=w563:errorcluster)  [unwired: 2 in]
                        n435 = Write to Binary File(file (use dialog)=w569, data=w556, error in=w567, 5:FALSE ("prepend array or string size? (T)")) -> (refnum out=w568:refnum<file>, error out=w566:errorcluster)  [unwired: 2 in, 1 out]
                        n436 = Write to Binary File(file (use dialog)=w565, data=w553, error in=w563, 5:FALSE ("prepend array or string size? (T)")) -> (refnum out=w564:refnum<file>, error out=w562:errorcluster)  [unwired: 2 in, 1 out]
                        n437 = Get File Position(4:w566, 7:w568) -> (2:w559:i64)  [unwired: 2 out]
                        n438 = Get File Position(4:w562, 7:w564) -> (2:w552:i64)  [unwired: 2 out]
                        n439 = local write "FF_Off_Ptr"(w559) -> ()
                        n440 = local write "NF_Off_Ptr"(w552) -> ()
                      }
                    }
                  }
                }
              }
              frame #4 {
                n441 = First Call?() -> (First Call?: T/F=w581:bool)
                n442 = Or(x="calculate absorption cross sections", y=w581) -> (x .or. y?=w579:bool)
                n443 = case shown="True" w579 {
                  frame False {
                  }
                  frame True {
                    # "calculate absorption cross sections from HITRAN data base"
                    n444 = local read "Off-Line Smoothed"() -> (w582:dbl[])
                    n445 = local read "Lambda On Read (nm)"() -> (w585:dbl)
                    n446 = local read "Lambda Off Set (nm)"() -> (w588:dbl)
                    n447 = local read "Temperature (C)"() -> (w586:dbl)
                    n448 = local read "Pressure (mb)"() -> (w587:dbl)
                    n449 = script code="%Importing HITRAN data\n%hitran = dlmread('C:\\Users\\H2ODial\\Desktop\\Shared Telescope WV DIAL Code\\Libraries and VIs\\824nm_841nm_H2O.csv', ',',[0 1 352 7]);\nhitran = dlmread('C:\\Users\\H2ODial\\Desktop\\Shared Telescope WV DIAL Code\\Libraries and VIs\\824nm_841nm_H2O_Spectral_Calc.csv', ',',[1 1 1209 7]);\n\n%Range vector in meters\nrange = ([75:75:size(Online,2)*75]);\n\nif lambda< 828\nlambda=828.195;\nelse\nlambda=lambda;\nend;\n\n%%\n\n%Voigt profile calculation\nWNmin = 12070.0;\nWNmax = 12076.0;\n\n%Find lines from WNmin to WNmax to calculate voigt profile\nline_indices = find(hitran(1:size(hitran,1),1)>WNmin & hitran(1:size(hitran,1),1)<WNmax);\n\nline = (hitran(line_indices, 1:size(hitran,2)));\n\n%Calculate temperature and pressure profile\nT0 = 273+15.6;\nT0 = 273+T0_C;\n\nT = T0-0.005545.*range; \n\nP0  = 1.0;\nP0  = P0_mb/1000*0.986; %pressure in mb converted to atm\n\nP = P0.*(T0./T).^-5.21986;\n\n%linewidth temperature dependence factor\nalpha = line(:,7);        \n\n%initial Lorentz linewidth from HiTRAN [cm^-1]\ngammal0 = line(:,4);     \n\n%ground state transition energy [cm^-1]\nE = line(:,6);           \n\n%initial linestrength from HiTRAN [cm^-1/(mol*cm^-2)]\nS0 = line(:,2);      \n\n%absorption line center wavenumber from HiTRAN [cm^-1]\nnu0_0 = line(:,1);    \n\nnu_on = (1/(lambda)*1e7);\n\nnu_off = (1/(lambda_off)*1e7);\n\n\nfor i = 1:size(Online,2);\n\n    %Pressure shift\n    nu0 = nu0_0-.0428.*P(i);\n    \n    %Calculate Lorentz lineweidth at temperature T [cm^-1]\n    gammal = gammal0.*(P(i)./P0).*((T0./T(i)).^alpha);\n    \n    %Calculate Doppler linewidth at temperature T [cm^-1]\n    gammad = (nu0).*((2.0.*1.38E-23.*T(i).*log(2.0))./(0.018.*3.0E8.*3.0E8./6.022E23)).^(0.5);\n    \n    y = (gammal./gammad).*((log(2.0)).^(0.5));\n    \n    x_on = ((nu_on-nu0)./gammad).*(log(2.0)).^(0.5);\n    \n    x_off = ((nu_off-nu0)./gammad).*(log(2.0)).^(0.5);\n    \n    %setting up Voigt convolution\n    stepsize = 1;\n    \n    t = [-200:1:199].*stepsize;\n    \n    t = repmat(t',1,length(x_on))';\n    \n    x_on = repmat(x_on,1,length(t));\n    \n    x_off = repmat(x_off,1,length(t));\n    \n    y = repmat(y,1,length(t));\n    \n    f_on = (exp(-t.^2.0))./(y.^2.0+(x_on-t).^2.0);\n    \n    f_off = (exp(-t.^2.0))./(y.^2.0+(x_off-t).^2.0);\n    \n    %Set the integration sum to zero to start\n    integral_on = 0.0;\n    \n    integral_off = 0.0;\n    \n    %Voigt integration\n    z_on = trapz(t(1,:),f_on,2);\n    \n    z_off =  trapz(t(1,:),f_off,2);\n    \n    integral_on = z_on;\n    \n    integral_off = z_off;\n    \n    %Calculate linestrength at temperature T\n    S = S0.*((T0./T(i)).^(1.5)).*exp(1.439.*E.*((1./T0)-(1./T(i))));\n    \n    %Calculate Doppler line-center cross section [cm^2]\n    K = (S./gammad).*(((log(2.0))./pi).^(0.5));\n    \n    %Calculate the Voigt profile\n    V_on = (y(1)/pi).*integral_on;\n    \n    V_off = (y(1)./pi).*integral_off;\n    \n    %Calculate the Voigt profile absorption cross section [cm^2]\n    sigmav_on = K.*V_on;\n    \n    sigmav_off = K.*V_off;\n    \n    %Sum contributions from all of the surrounding lines\n    sigma_on_total(i) = sum(sigmav_on);\n    \n    sigma_off_total(i) = sum(sigmav_off);\n    \nend;"("lambda"=w585, "lambda_off"=w588, "P0_mb"=w587, "T0_C"=w586, "Online"=w582) -> ("sigma_on_total"=→"sigma_on_total":dbl[], "sigma_off_total"=→"sigma_off_total":dbl[])  [unwired: 1 in, 1 out]
                  }
                }
              }
              frame #5 {
                w599 = 1
                # "normalization factor\nfrom 300 to 450m"
                # "OPTICAL DEPTH PLOT"
                # "new rainbow color bar display"
                # "Data Processing Far Channel"
                # "new rainbow color bar display"
                # "Calculating the range resolved water vapor number density and plotting"
                n450 = local read "sigma_off_total"() -> (w622:dbl[])
                n451 = local read "sigma_on_total"() -> (w619:dbl[])
                n452 = local read "On-Line  Smoothed"() -> (w597:dbl[])
                n453 = local read "Off-Line Smoothed"() -> (w596:dbl[])
                n454 = local read "Off-Line Smoothed 2"() -> (w620:dbl[])
                n455 = local read "On-Line Smoothed 2"() -> (w621:dbl[])
                n456 = script code="%Time averaging in seconds.  600 Seconds =10 minutes\ntemporal_average = 600;\n\n%Spatial averaging in bins.  2 bins = 150 meters\nspatial_average = 2;\n\n%Creating r and r+deltar vectors..this can also be acsomplished using the\n%diff command\np_oni = Online(:,1:size(Online,2)-1);\n\np_onii = Online(:,2:size(Online,2));\n\np_offi = Offline(:,1:size(Offline,2)-1);\n\np_offii = Offline(:,2:size(Offline,2));\n\nInside = (p_oni.*p_offii)./(p_onii.*p_offi);\n\ndel_cross = 1./(2.*(sigma_on_total(1:size(Online,2)-1)-sigma_off_total(1:size(Offline,2)-1)).*75*100);\n\ndel_cross(isinf(del_cross)) = 0;\n\n%Calculating Number density\nN = del_cross.*log(Inside);\n\n%Spatial smoothing of the profiles\nfilter1 = ones(1,2)./2;\n\nN_1 = N;\n\nN_1_avg = filter2(filter1,N_1);\n\nfilter1 = ones(1,10)./10;\n\nN_2 = N;\n\nN_2_avg = filter2(filter1,N_2);\n\nN_new = zeros(size(N,1),size(N,2));\n \n%Using different averaging windows for different altitudes \nN_avg=[N_1_avg(:,1:40)';N_2_avg(:,41:size(N,2))']';\n\n\nw = N_avg.*1e6.*18.015./6.022e23"("Online"=w621, "Offline"=w620, "sigma_on_total"=w619, "sigma_off_total"=w622) -> ("N_avg"=w623:cdb[], "w"=w632:cdb[])  [unwired: 1 in, 1 out]
                n457 = script code="%Time averaging in seconds.  600 Seconds = 10 minutes\ntemporal_average = 600;\n\n%Spatial averaging in bins.  2 bins = 150 meters\nspatial_average = 2;\n\n%Creating r and r+deltar vectors..this can also be acsomplished using the\n%diff command\np_oni = Online(:,1:size(Online,2)-1);\n\np_onii = Online(:,2:size(Online,2));\n\np_offi = Offline(:,1:size(Offline,2)-1);\n\np_offii = Offline(:,2:size(Offline,2));\n\nInside = (p_oni.*p_offii)./(p_onii.*p_offi);\n\ndel_cross = 1./(2.*(sigma_on_total(1:size(Online,2)-1)-sigma_off_total(1:size(Offline,2)-1)).*75*100);\n\ndel_cross(isinf(del_cross)) = 0;\n\n%Calculating Number density\nN = del_cross.*log(Inside);\n\n%Spatial smoothing of the profiles\nfilter1 = ones(1,2)./2;\n\nN_1 = N;\n\nN_1_avg = filter2(filter1,N_1);\n\nfilter1 = ones(1,10)./10;\n\nN_2 = N;\n\nN_2_avg = filter2(filter1,N_2);\n\nN_new = zeros(size(N,1),size(N,2));\n \n%Using different averaging windows for different altitudes \nN_avg=[N_1_avg(:,1:40)';N_2_avg(:,41:size(N,2))']';\n\n \nw = N_avg.*1e6.*18.015./6.022e23"("Online"=w597, "Offline"=w596, "sigma_on_total"=w619, "sigma_off_total"=w622) -> ("N_avg"=w628:cdb[], "w"=w629:cdb[])  [unwired: 1 in, 1 out]
                n458 = local read "Time Resolution Per Bin(ns)"() -> (w598:u32)
                n459 = local read "bins"() -> (w624:u32)
                n460 = local read "Altitude Array (km)"() -> (w594:dbl[])
                n461 = Build Array(w629, w632) -> (w635:cdb[][])
                n462 = To Double Precision Float(number=w598) -> (double precision float=w617:dbl)
                n463 = Reshape Array(w628, w599, w624) -> (w639:cdb[][])
                n464 = Reshape Array(w623, w599, w624) -> (w626:cdb[][])
                n465 = Multiply(x=0.15, y=w617) -> (x*y=w615:dbl)
                n466 = Build Array(w628, w623) -> (w633:cdb[][])
                n467 = Divide(x=300.0, y=w615) -> (x/y=w612:dbl)
                n468 = Divide(x=450.0, y=w615) -> (x/y=w611:dbl)
                n469 = Build Array(w594, w594) -> (w618:dbl[][])
                n470 = call "Convert to Dynamic Data5"("2D Array"=w635) -> ("Dynamic Data Type"=w634:dynamicdata)  [unwired: 3 in]
                n471 = call "Convert to Dynamic Data2"("2D Array"=w633) -> ("Dynamic Data Type"=w630:dynamicdata)  [unwired: 3 in]
                n472 = Divide(x=w639, y=1e+17) -> (x/y=→"Water Vapor Number Density":cdb[][])
                n473 = Divide(x=w626, y=1e+17) -> (x/y=→"Water Vapor Number Density 2":cdb[][])
                n474 = call "Convert to Dynamic Data6"("Array"=w594) -> ("Dynamic Data Type"=w595:dynamicdata)  [unwired: 3 in]
                n475 = To Long Integer(number=w612) -> (32bit integer=w610:i32)
                n476 = To Long Integer(number=w611) -> (32bit integer=w609:i32)
                n477 = call "Convert to Dynamic Data"("2D Array"=w618) -> ("Dynamic Data Type"=w631:dynamicdata)  [unwired: 3 in]
                n478 = call "Convert to Dynamic Data8"("2D Array"=w618) -> ("Dynamic Data Type"=w636:dynamicdata)  [unwired: 3 in]
                n479 = Decrement(x=w610) -> (x-1=w607:i32)
                n480 = Decrement(x=w609) -> (x-1=w608:i32)
                n481 = call "Build XY Graph"("Y Input"=w631, "X Input"=w630) -> ("XY Graph"=→"Water Vapor Number Density  2":cluster{"Y":dbl[], "Y":dbl[]}[])  [unwired: 3 in, 6 out]
                n482 = call "Build XY Graph3"("Y Input"=w636, "X Input"=w634) -> ("XY Graph"=→"Absolute Humidity":cluster{"Y":dbl[], "Y":dbl[]}[])  [unwired: 3 in, 6 out]
                n483 = Array Subset(array=w597, index=w607, length=w608) -> (w606:dbl[])
                n484 = Array Subset(array=w596, index=w607, length=w608) -> (w605:dbl[])
                n485 = call-poly <vilib>:"Mean.vi"("X"=w606) -> ("mean"=w604:dbl)  [unwired: 1 out]
                n486 = call-poly <vilib>:"Mean.vi"("X"=w605) -> ("mean"=w603:dbl)  [unwired: 1 out]
                n487 = Divide(x=w604, y=w603) -> (x/y=w602:dbl)
                n488 = Multiply(x=w596, y=w602) -> (x*y=w601:dbl[])
                n489 = Divide(x=w597, y=w601) -> (x/y=w600:dbl[])
                n490 = Natural Logarithm(1:w600) -> (0:w591:dbl[])
                n491 = Multiply(x=-1.0, y=w591) -> (x*y=w590:dbl[])
                n492 = call "Convert to Dynamic Data9"("Array"=w590) -> ("Dynamic Data Type"=w593:dynamicdata)  [unwired: 3 in]
                n493 = call "Build OD Plot"("Y Input"=w595, "X Input"=w593) -> ("XY Graph"=→"Optical Depth":cluster{"Y":dbl[], "Y":dbl[]}[])  [unwired: 3 in, 6 out]
              }
            }
          }
        }
        "L_Count" <- w126
      }
    }
  }
  n494 = case shown="True" w3 {
    frame False {
    }
    frame True {
      # "close data files"
      n495 = local read "NF_Off_Ref"() -> (w642:refnum<file>)
      n496 = local read "NF_On_Ref"() -> (w643:refnum<file>)
      n497 = local read "FF_Off_Ref"() -> (w644:refnum<file>)
      n498 = local read "FF_On_Ref"() -> (w645:refnum<file>)
      n499 = Close File(refnum=w645) -> ()  [unwired: 1 in, 2 out]
      n500 = Close File(refnum=w644) -> ()  [unwired: 1 in, 2 out]
      n501 = Close File(refnum=w643) -> ()  [unwired: 1 in, 2 out]
      n502 = Close File(refnum=w642) -> ()  [unwired: 1 in, 2 out]
    }
  }
  "FileHour" <- -1 ("FileHour")
  "DataOpen" <- FALSE
